vi "main.vi"() -> ()   [LabVIEW 2020]
uses:
  measure/Meas Session.ctl
  adc/ADC Session.ctl
  drivers/niScope/niScope Session.ctl
  drivers/niScope/niScope Virtual Channel Config.ctl
  drivers/niScope/niScope Virtual Channel Mode.ctl
  drivers/niScope/niScope Virtual Channel Input Z.ctl
  drivers/niScope/niScope Virtual Channel Coupling.ctl
  drivers/niScope/niScope Type.ctl
  drivers/niScope/niScope Digitizing Process Options.ctl
  drivers/niScope/niScope Data Packet.ctl
  drivers/niScope/niScope Trigger Setup.ctl
  <instrlib>/niScope/Controls/niScope trigger coupling.ctl
  <instrlib>/niScope/Controls/niScope trigger slope.ctl
  drivers/niScope/niScope Reference Clock.ctl
  drivers/DMM/3458A Digitizer Session.ctl
  drivers/DMM/3458A Virtual Channel Config.ctl
  drivers/Counter/Counter Session.ctl
  drivers/Counter/Counter Type.ctl
  drivers/AWG/AWG Session.ctl
  drivers/AWG/AWG Type.ctl
  drivers/AWG/CMI Clock Divider v2/CMI ckd2 Session.ctl
  drivers/AWG/CMI Clock Divider v2/CMI ckd2 Source Mode.ctl
  drivers/AWG/CMI Clock Divider v2/CMI ckd2 Divisor Mode.ctl
  drivers/AWG/CMI Sync V3/CMI Sync V3 session.ctl
  drivers/AWG/CMI Sync V3/Configure/CMI Sync V3 Reference Clock Source.ctl
  drivers/AWG/CMI Sync V3/Configure/CMI Sync V3 HV input Range.ctl
  drivers/AWG/CMI Sync V3/Configure/CMI Sync V3 Trigger Input Level.ctl
  drivers/AWG/CMI Sync V3/Configure/CMI Sync V3 Channel 1 Mode.ctl
  drivers/AWG/CMI Sync V3/Configure/CMI Sync V3 Channel Output Levels.ctl
  drivers/AWG/CMI Sync V3/Configure/CMI Sync V3 Channel 2 Mode.ctl
  drivers/AWG/CMI Sync V3/Configure/CMI Sync V3 Channel 3 Mode.ctl
  drivers/AWG/CMI Sync V3/Configure/CMI Sync V3 Channel 1 Divisor Entry Mode.ctl
  adc/ADC Trig Config.ctl
  adc/ADC Trig Mode Source.ctl
  adc/ADC Trig Slope.ctl
  adc/ADC Trig Coupling.ctl
  drivers/AWG/RaS HMF2500/HMF2500 Config.ctl
  drivers/DMM/3458A Sync Mode.ctl
  drivers/DMM/3458A Idn Mode.ctl
  drivers/DMM/3458A Digitizing Low Levels/Configure/Sampling Mode.ctl
  drivers/DMM/3458A Digitizing Process Options.ctl
  drivers/DMM/3458A Data Packet.ctl
  drivers/DMM/3458A Aux Record Data.ctl
  drivers/DMM/3458A Digitizing Low Levels/Configure/Level Setup.ctl
  drivers/DMM/3458A Digitizing Low Levels/Configure/First Sample Trigger.ctl
  drivers/DMM/3458A Aperture Selection Mode.ctl
  drivers/DMM/3458A Multiplexing Config.ctl
  drivers/Fluke 8588A/F8588A Low Pass Filter.ctl
  drivers/Fluke 8588A/F8588A Phase Lock.ctl
  drivers/Fluke 8588A/F8588A Coupling.ctl
  drivers/DMM/3458A Sampling Rate.ctl
  drivers/AWG/AWG Clock Setup Mode.ctl
  drivers/DMM/3458A Sample Rate Mode.ctl
  drivers/dsdll/DSDLL Session.ctl
  drivers/dsdll/dsdll/dsdll_instance.ctl
  drivers/dsdll/dsdll/dsdll_device_record.ctl
  drivers/dsdll/DSDLL Process Config.ctl
  drivers/dsdll/DSDLL Data Packet.ctl
  adc/ADC Type.ctl
  drivers/simulated_adc/SimAdc Config.ctl
  drivers/simulated_adc/SimAdc Channel Cfg.ctl
  adc/ADC On Close Action.ctl
  adc/Multiplexer/MPX Session.ctl
  adc/Multiplexer/MPX Type.ctl
  drivers/Multiplexers/Generic COM/GCOMM Session.ctl
  drivers/Multiplexers/Generic COM/GCOMM Signal.ctl
  drivers/Multiplexers/Generic COM/GCOMM Virtual Channel.ctl
  drivers/Multiplexers/Generic COM/GCOMM Logic State.ctl
  drivers/Multiplexers/Generic COM/QPMX Session.ctl
  drivers/Multiplexers/QPMX/QPMX switch mode.ctl
  drivers/Multiplexers/QPMX/QPMX polarity.ctl
  drivers/Multiplexers/Generic VISA commands/GVISA Mux Session.ctl
  drivers/Multiplexers/Generic VISA commands/GVISA Mux Path Entry.ctl
  drivers/Multiplexers/Generic VISA commands/met_serial_setup.ctl
  drivers/Agilent DSO 90000/Virtual Digitizer/KeDSO session.ctl
  drivers/Agilent DSO 90000/Virtual Digitizer/KeDSO Virtual Channel.ctl
  drivers/Agilent DSO 90000/Virtual Digitizer/KeDSO High Resolution Mode.ctl
  drivers/Agilent DSO 90000/Virtual Digitizer/KeDSO Trigger Setup.ctl
  drivers/Agilent DSO 90000/Virtual Digitizer/KeDSO Trigger Source.ctl
  drivers/Agilent DSO 90000/Public/Utility/DSO type.ctl
  drivers/cdaq/cDAQ Session.ctl
  drivers/cdaq/low_level_old/cdaq_anal_adc_command.ctl
  drivers/cdaq/low_level_old/cdaq_anal_adc_data.ctl
  drivers/cdaq/cDAQ Virtual Channel.ctl
  drivers/cdaq/cDAQ Master Clock Mode.ctl
  measure/Meas Sequence Item.ctl
  measure/Meas Sampling Configuration.ctl
  measure/processing/QWTB/Meas Proc QWTB Algorithm Parameter Data.ctl
  measure/Meas Sequence Configuration.ctl
  measure/Meas Range Mode.ctl
  measure/Meas Sampling Rate Mode.ctl
  octave/golpi/mpc/golpi_session_ref.ctl
  octave/golpi/mpc/golpi_session.ctl
  octave/golpi/GOLPI reference Type Def.ctl
  octave/golpi/Pipe Handle.ctl
  measure/processing/Meas Process Config.ctl
  measure/processing/Meas Process Mode.ctl
  measure/processing/Meas Process Raw Config.ctl
  measure/processing/Meas Process Raw Result Mode.ctl
  measure/processing/QWTB/Meas Proc QWTB Setup.ctl
  measure/processing/QWTB/Meas Proc QWTB Uncertainty Mode.ctl
  measure/processing/QWTB/Meas Proc QWTB Multicore Setup.ctl
  measure/processing/QWTB/Meas Proc QWTB Multicore Type.ctl
  measure/processing/Meas Process Time Stamp Mode.ctl
  measure/processing/QWTB/Meas Proc QWTB Exec Mode.ctl
  measure/Corrections/Corr Setup.ctl
  measure/Corrections/Corr Tranducer Item.ctl
  measure/Corrections/Corr Digitizers.ctl
  measure/Assist/Assist Panel Setup.ctl
  measure/processing/QWTB/Meas Proc QWTB View Max Dim.ctl
  measure/processing/QWTB/Meas Proc QWTB View Uncertainty Mode.ctl
  measure/processing/QWTB/Meas Proc QWTB View Group Mode.ctl
  measure/processing/QWTB/Meas Proc QWTB Viewer References.ctl
  measure/processing/QWTB/Meas Proc QWTB View Phase Mode.ctl
  measure/processing/QWTB/Meas Proc QWTB View Amplitude Mode.ctl
  server/Server Event GUI command.ctl
  server/Server Session.ctl
  varilib/SGUI Assign References Mode.ctl
  server/Server Event.ctl
  server/Server Client Request.ctl
  server/Server Event Command.ctl
  <vilib>/Utility/miscctls.llb/LVRowAndColumnTypeDef.ctl
  varilib/SGUI Assign Multiple Strings With Tags By Label.vi
  varilib/varilib.lvlib
  drivers/niScope/niScope Virtual Digitizer.lvlib
  drivers/DMM/3458A Virtual Digitizer.lvlib
  drivers/Counter/Counter.lvlib
  drivers/AWG/AWG.lvlib
  drivers/DMM/3458A Digitizing Low Levels/3458A Digitizing Low Levels.lvlib
  drivers/dsdll/DSDLL Virtual Digitizer.lvlib
  octave/golpi/mpc/GOLPI Multi Process.lvlib
  drivers/dsdll/dsdll/dsdll.lvlib
  drivers/AWG/CMI Sync V3/CMI Sync Unit V3.lvlib
  drivers/Agilent DSO 90000/Agilent 90000 Series.lvlib
  octave/golpi/GOLPI library.lvlib
  octave/golpi/LV Process library.lvlib
panel:
  out "stat4":string
  in  "btn view fft":bool
  in  "server":T1
  out "start btns":T2
  in  "server vi ref":refnum<vi>
  in  "btn srv":bool
  in  "btn qwtb calc":bool
  in  "qwtb view VI ref":refnum<vi>
  in  "exp tab":string[][](table)
  in  "btn about":bool
  out "qwtb view":T3
  in  "tc result":enum32{"RAW", "QWTB"}(tab)=enum."QWTB"
  out "str res":string caption="Result"
  in  "qwtb comment":string caption="Note:"
  in  "qwtb amp":T4 caption="Convert amplitude"
  out "qwtb meas pth":string caption="Selected measurement:"
  in  "qwtb alg sel":u16(ring) caption="Algorithm selection" items=["Current: TWM-PWRTDI", "TWM-PWRTDI"]
  in  "qwtb meas sel":u16(ring) caption="Measurement selection" items=["None", "Current", "Load from file"]
  in  "qwtb ref chn":u16(ring) caption="Ref. channel" items=["None", "L1"]
  in  "qwtb ph unit":T5 caption="Phase mode"
  out "qwtb res info":string caption="Info:"
  in  "qwtb res sel":u16(ring) caption="Result selection" items=["Current result", "Average", "RESULTS\\TWM-PWRTDI-G0001-A0001"]
  in  "qwtb maxarr":i32=10 caption="Max shown array size" min=1 max=1000 step=1
  in  "qwtb order":T6 caption="Res. order mode"
  in  "qwtb unc":T7 caption="Uncertainty display"
  in  "qwtb maxdim":T8 caption="Max. shown dimension"
  out "qwtb results table":string[][](table) caption="Results (right click to table to show actions)"
  in  "qwtb qu list":i32[](listbox) caption="Select quantities"
  in  "qwtb save comment":bool
  in  "btn set&start":bool
  in  "btn setup":bool
  in  "btn corr":bool
  in  "btn view rec":bool
  in  "golpi":T9={"GOLPI ref"={"pipe handle"={"lv_proc.dll file path"=path "", "process instance handle"=[], "debug mode"=FALSE, "debug data"=[]}, "fast read timeout [ms]"=500, "fast read settle time [ms]"=10, "fast read to multiple [ms]"=1, "max elements per input line"=100, "slow read timeout [ms]"=5000, "stdin double format specifier"="%_16e", "max elements per stdout output column"=100, "console mode bitstream"=FALSE, "bitstream first read timeout [ms]"=1000, "bitstream read timeout [ms]"=50, "struct transfer possible"=FALSE, "matlab mode"=FALSE}, "idn str"="", "octave path"=path "C:/Octave364/Octave3.6.4_gcc4.6.2/bin", "work path"=path "C:/Octave364/Octave3.6.4_gcc4.6.2/bin", "start timeout [ms]"=15000, "clr cache"=FALSE, "console"=FALSE, "binary"=FALSE, "semaphore"=refnum, "initial command"="", "exit command"="", "matlab"=FALSE, "pkg list"=[]}
  out "stat3":string
  out "stat2":string
  in  "session VI ref":refnum<vi>
  out "stat1":string
  in  "session":T13={"adc"={"niScope"={"channel cfg"=[], "sessions"=[], "multi cards"=FALSE, "channels"=0, "type"=enum."n/a", "memory [B/chn]"=0, "ext. clock [Hz]"=0.0, "samples count"=0, "use streaming"=FALSE, "proc setup"={"packet size [smpl]"=0, "current timeout [s]"=0.0, "blk2blk timeout [s]"=0.0, "event time"=timestamp(0 s since 1904-01-01), "temp sampl T [s]"=0.0, "data queue"=refnum, "stop notifier"=refnum, "proc ref"=refnum}, "sample width [B]"=0, "ranges [V]"=[], "trigger setup"={"coupling"=1, "level [V]"=0.0, "slope"=0, "mode"=enum."Immediate", "pre-trigger [%]"=0.0}, "fs [Hz]"=0.0, "bitres [bit]"=0, "clock source"=enum."VAL_NO_SOURCE"}, "3458A"={"channels"=[], "sync unit"={"VISA"="", "type"=enum."Picotest U6200A"}, "awg unit"={"type"=enum."Agilent 331xxA to 332xxA", "VISA"="", "enable 10MHz ref"=FALSE, "cmi ckd2"={"VISA"="", "clock source"=enum."Auto", "manual ref clk"=FALSE, "ref clock [Hz]"=0.0, "div mode"=enum."Set divisor directly"}, "cmi sync v3"={"VISA"="", "baud rate [bd/s]"=115200, "source"=enum."Auto", "hv range"=enum."1kV", "fsrc is fixed"=FALSE, "fsrc [Hz]"=10000000.0, "freq integ [s]"=1.0, "freq filter"=5, "trig level"=enum."TTL 5V", "chn1 mode"=enum."Source divider", "chn1 level"=enum."Positive 5V", "chn2 mode"=enum."Source divider", "chn2 level"=enum."Positive 5V", "chn2 div"=1, "chn3 mode"=enum."Chn 1 Active", "chn3 level"=enum."Positive 5V", "chn1 div entry"=enum."Calculate nearest divisor from measured fx", "chn1 dev limit [%]"=1.0, "chn1 check dev"=FALSE}, "trigger"={"source"=enum."Immediate", "slope"=enum."POS", "coupling"=enum."DC", "level [V]"=0.0, "hysteresis [V]"=0.0, "pre-trigger [%]"=0.0}, "HMF2500 cfg"={"Baud Rate"=9600, "Parity"=0, "Data Bits"=8, "Flow Control"=4}}, "sync mode"=enum."MASTER-SLAVE, MASTER clocked by TIMER", "streaming mode"=FALSE, "idn mode"=enum."Auto", "sampling mode"=enum."DCV", "sample memory [B]"=0, "proc setup"={"channel id"=0, "packet size [smpl]"=0, "current timeout [s]"=0.0, "blk2blk timeout [s]"=0.0, "event time"=timestamp(0 s since 1904-01-01), "stop notifier"=refnum, "data queues"=[], "proc refs"=[], "bus semaphore"=refnum}, "sample size [B]"=0, "sample count"=0, "aux data"={"channel id"=0, "valid?"=[], "gain [V]"=[], "timestamp [s]"=[], "Ts [s]"=0.0, "abs timestamp"=timestamp(0 s since 1904-01-01), "t [deg C]"=[], "multiplex timestamp [s]"=-1.0, "only multiplex?"=FALSE, "multiplex smpl offset"=0, "overflow?"=FALSE}, "ranges [V]"=[], "aperture [s]"=0.0, "LEVEL trigger"={"edge"=enum."POS", "level [V]"=0.0, "coupling"=enum."DC"}, "trigger mode"=enum."AUTO", "measure temp.?"=FALSE, "disp mesages"=[], "shared bus?"=FALSE, "disable display?"=FALSE, "aper mode"=enum."Manual", "aper rules"=[], "multiplex"={"cycles"=0, "delay [s]"=0.0, "enabled"=FALSE, "overhead [s]"=1.0, "tot smpls"=0, "sub-rec"=0, "overhead [%]"=0.0, "emulated"=FALSE}, "F8588 lpf"=enum."Off", "F8588 pll"=enum."Off", "F8588 couple"=enum."DC, auto", "fs"={"freq mode"=enum."fs or Ts", "fs [Hz]"=0.0, "fref [Hz]"=0.0, "mul"=0.0, "div"=0.0}, "fs mode"=enum."fs or Ts"}, "dsdll"={"dsdll"={"dsdll path"=path "", "dsdll handle"=[], "output devices"=[], "capture devices"=[]}, "channels"=0, "device id"=0, "channel idns"=[], "proc setup"={"packet size [smpl]"=0, "current timeout [s]"=0.0, "blk2blk timeout [s]"=0.0, "event time"=timestamp(0 s since 1904-01-01), "data queue"=refnum, "stop notifier"=refnum, "proc ref"=refnum}, "samples count"=0, "fs [Hz]"=0.0}, "type"=enum."niScope", "channel idn str"=[], "aux instr idn str"=[], "modified?"=FALSE, "simadc"={"channels"=[], "range [V]"=0.0, "Ts step [s]"=0.0, "time [s]"=0.0, "fs [Hz]"=0.0, "count"=0, "smpl offset"=0, "set count"=0, "bit res"=0}, "force rst?"=FALSE, "exit mode"=enum."Immediate reset", "exit dly"=0.0, "exit tmr"=timestamp(0 s since 1904-01-01), "busy?"=FALSE, "accessed?"=FALSE, "multiplex"={"Type"=enum."Dummy", "gen com ssn"={"visa"="", "primary"=enum."None", "secondary"=enum."None", "channels"=[]}, "delay before [s]"=0.0, "delay post [s]"=0.0, "sequence"=[], "enabled"=FALSE, "ref timestamp [s]"=0.0, "idn string"="", "dev niScope"="", "niScope idx"=0, "QPMX ssn"={"visa"="", "switch mode"=enum."Switched by TWM", "sequence"=[], "timing delays"=[], "polarity"=enum."Positive", "ss delay (s)"=2.0, "internal timer (s)"=1.0, "Last loaded sequence file"=path "", "startup delay (s)"=2.0}, "VISA mux ssn"={"VISA"="", "paths"=[], "idn command"="", "serial cfg"={"Baud rate"=9600, "Data bits"=8, "Parity"=0, "Stop bits"=10, "Flow control"=0, "End Mode Read"=enum."None", "End Mode Write"=enum."None", "Term character"=0, "Term enable"=FALSE}}}, "keysight dso"={"VISA"="", "channels"=[], "bw limit [Hz]"=0.0, "resolution"=enum."Basic", "trig noise reject"=enum."Normal", "N"=0, "trigger config"={"trigger source"=enum."Immediate", "trigger slope"=enum."Negative", "level [V]"=0.0, "hysteresis [V]"=0.001, "pre-trig [%]"=50}, "fs [Hz]"=0.0, "timeout stop"=timestamp(0 s since 1904-01-01), "waiting for opc"=FALSE, "fetch offset [smpl]"=0, "abs timestamp"=timestamp(0 s since 1904-01-01), "ranges [V]"=[], "decimation"=1.0, "ext ref"=FALSE, "emulate aperture"=FALSE, "model"=enum."DSO91304"}, "cdaq"={"mclk [Hz]"=12800000.0, "ADC task"="", "mclk reference"="", "fs [Hz]"=50000.0, "queue adc cmd"=refnum, "queue adc data"=refnum, "adc proc ref"=refnum, "channels"=[], "last channels"=[], "timeout"=timestamp(0 s since 1904-01-01), "N"=1000, "mclk mode"=enum."Free running", "ext mclk source"=""}, "ignore overload"=FALSE}, "sequence"=[], "sequence setup"={"group setups"=[], "rec count"=0, "range mode"=enum."Keep defaults", "fs mode"=enum."Frequency", "rng even"=0.0, "rng odd"=0.0, "folder"=path "", "name base"="", "meas id"=0, "settle [s]"=0.0, "comment"="", "avg count"=0, "fs-abs-fr fr"=0.0, "fs-abs-fr fs"=0.0, "fs-div fr"=0.0, "fs-div div"=0.0, "fs-mn fr"=0.0, "fs-mn mul"=0.0, "fs-mn div"=0.0, "fs-rat fr"=0.0, "fs-rat rat"=0.0}, "golpi"=refnum, "processing setup"={"mode"=enum."Raw", "call after avgs?"=FALSE, "calculate?"=FALSE, "raw mode"={"command"="", "result mode"=enum."Display console output (only Octave)", "res variable"=""}, "QWTB"={"QWTB path"=path "", "alg filter path"="", "alg ids"=[], "alg parameters"=[], "parsed parameters"=[], "selected alg id"="", "selected unc mode"=enum."None", "qwtb mcc"=100, "qwtb timeout"=90, "qwtb covg"=95.0, "qwtb ofs"=0, "qwtb lim data"=0, "multicore"={"jobs folder"=path "", "cores"=0, "max jobs"=0, "mode"=enum."Singlecore"}, "unc once?"=FALSE, "qwtb tstemp"=enum."Enabled (default)", "octave reset"=FALSE, "exec mode"=enum."Single-core"}}, "corrections"={"transducers"={"channels"=[], "last path"=path "", "root path"=path ""}, "digitizer"={"last path"=path "", "channel paths"=[], "channel idns"=[], "correction name"="", "channel names"=[], "folders to copy"=[], "channel valid"=[], "correction path"=path "", "correction rel path"="", "rel folders to copy"=[], "root path"=path ""}}, "assist cfg"={"P"=0, "Q"=0, "rel shift"=0.0, "ref freq"=0.0, "min fs"=0.0, "max fs tol"=0.0, "min int"=0.0, "max int"=0.0, "max err"=0.0, "max timeout"=0.0}} {"corrections"."transducers"."channels"."Phase index" min=1 step=1; "adc"."cdaq"."last channels"."Channel id" min=0 step=1; "adc"."cdaq"."channels"."Channel id" min=0 step=1; "adc"."keysight dso"."decimation" min=1.0; "adc"."keysight dso"."bw limit [Hz]" format="%#_6p"; "adc"."keysight dso"."channels"."Offset [V]" format="%#_6p"; "adc"."keysight dso"."channels"."Range [Vpk]" min=0.0 format="%#_6p"; "adc"."keysight dso"."channels"."Channel" min=1; "adc"."multiplex"."VISA mux ssn"."serial cfg"."Flow control" items=["None", "XON/XOFF", "CTS/RTS", "XON/XOFF + CTS/RTS", "DTR/DSR", "XON/XOFF + DTR/DSR"]; "adc"."multiplex"."VISA mux ssn"."serial cfg"."Stop bits" items=["1 bit"=10, "1.5 bits"=15, "2 bits"=20]; "adc"."multiplex"."VISA mux ssn"."serial cfg"."Parity" items=["None", "Odd", "Even", "Mark", "Space"]; "adc"."multiplex"."VISA mux ssn"."serial cfg"."Data bits" items=["5 bits"=5, "6 bits"=6, "7 bits"=7, "8 bits"=8]; "adc"."multiplex"."VISA mux ssn"."serial cfg"."Baud rate" items=["150 Bd"=150, "300 Bd"=300, "600 Bd"=600, "1200 Bd"=1200, "2400 Bd"=2400, "4800 Bd"=4800, "9600 Bd"=9600, "19.2 kBd"=19200, "38.4 kBd"=38400, "57.6 kBd"=57600, "115.2 kBd"=115200]; "adc"."multiplex"."QPMX ssn"."startup delay (s)" min=0.0 step=1.0; "adc"."multiplex"."QPMX ssn"."internal timer (s)" min=0.0 step=1.0; "adc"."multiplex"."QPMX ssn"."ss delay (s)" min=0.0 step=1.0; "adc"."multiplex"."QPMX ssn"."timing delays" min=1 max=255 step=1; "adc"."3458A"."awg unit"."HMF2500 cfg"."Flow Control" items=["None", "XON/XOFF", "RTS/CTS", "XON/XOFF & RTS/CTS", "DTR/DSR", "XON/XOFF & DTR/DSR"]; "adc"."3458A"."awg unit"."HMF2500 cfg"."Data Bits" items=["7"=7, "8"=8]; "adc"."3458A"."awg unit"."HMF2500 cfg"."Parity" items=["None", "Odd", "Even", "Mark", "Space"]; "adc"."3458A"."awg unit"."HMF2500 cfg"."Baud Rate" items=["300"=300, "600"=600, "1200"=1200, "2400"=2400, "4800"=4800, "9600"=9600, "19200"=19200]; "adc"."3458A"."awg unit"."cmi sync v3"."chn2 div" min=1 max=100000000 step=1; "adc"."3458A"."awg unit"."cmi sync v3"."fsrc [Hz]" format="%_8p"; "adc"."3458A"."channels"."Range [Vpk]" min=0.0; "adc"."niScope"."trigger setup"."pre-trigger [%]" format="%.2f"; "adc"."niScope"."trigger setup"."level [V]" format="%.2f"; "adc"."niScope"."trigger setup"."coupling" items=["AC"=0, "DC"=1, "HF Reject"=3, "LF Reject"=4, "AC Plus HF Reject"=1001]; "adc"."niScope"."channel cfg"."Range [Vpk]" min=0.0; "adc"."niScope"."channel cfg"."Channel" min=0}
  in  "btn stop":bool
  in  "btn start":bool
  out "error":errorcluster
  in  "btn exit":bool
  in  "btn cfg adc":bool
  in  "btn cfg octave":bool
  # "ADC:"
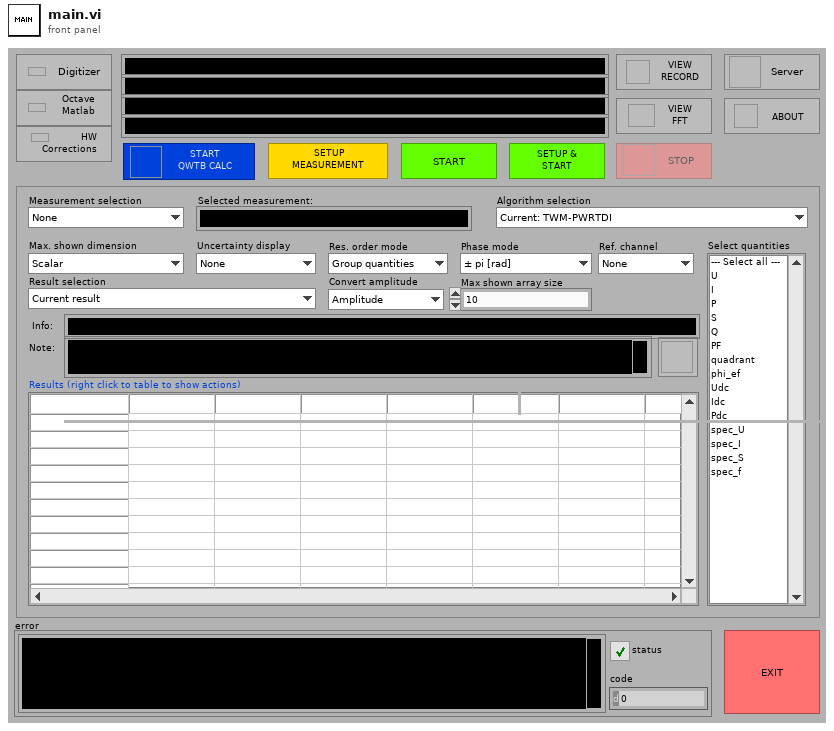
[diagram p1: front panel]
types:
  T1 = typedef "Server Session.ctl" = cluster{"cmd event":variant, "answer event":variant}
  T2 = typedef "Server Event GUI command.ctl" = cluster{"start":bool, "setup":bool, "setup&start":bool}
  T3 = typedef "Meas Proc QWTB Viewer References.ctl" = cluster{"tc result":refnum<vi>, "qwtb results tbl":refnum<vi>, "qwtb maxdim":refnum<vi>, "qwtb unc":refnum<vi>, "qwtb order":refnum<vi>, "qwtb maxarr":refnum<vi>, "qwtb res sel":refnum<vi>, "qwtb res info":refnum<vi>, "descriptions":string[], "var names":string[], "channel indexes":i32[], "qwtb ref chn":refnum<vi>, "qwtb ph unit":refnum<vi>, "qwtb alg sel":refnum<vi>, "qwtb meas sel":refnum<vi>, "qwtb ssn info":refnum<vi>, "last session (man)":path, "qwtb qu list":refnum<vi>, "matrix":dbl[][], "comment":string, "qwtb comment":refnum<vi>, "last session":path, "qwtb amp":refnum<vi>}
  T4 = typedef "Meas Proc QWTB View Amplitude Mode.ctl" = enum16{"Amplitude", "Effective", "amp. * sqrt(3)", "amp. / sqrt(3)", "eff. * sqrt(3)", "eff. / sqrt(3)", "Peak-Peak", "dB", "dBmV (dBmA)", "dBuV (dBuA)"}
  T5 = typedef "Meas Proc QWTB View Phase Mode.ctl" = enum16{"± pi [rad]", "0 - 2*pi [rad]", "±180 [deg]", "0 - 360 [deg]"}
  T6 = typedef "Meas Proc QWTB View Group Mode.ctl" = enum16{"Group quantities", "Group phases"}
  T7 = typedef "Meas Proc QWTB View Uncertainty Mode.ctl" = enum16{"None", "val ± unc", "[val; unc]"}
  T8 = typedef "Meas Proc QWTB View Max Dim.ctl" = enum16{"Scalar", "Vector", "Matrix"}
  T9 = typedef "GOLPI Multi Process.lvlib/golpi_session.ctl" = cluster{"GOLPI ref":T10, "idn str":string, "octave path":path, "work path":path, "start timeout [ms]":u32, "clr cache":bool, "console":bool, "binary":bool, "semaphore":T12, "initial command":string, "exit command":string, "matlab":bool, "pkg list":string[]}
  T10 = typedef "GOLPI library.lvlib/GOLPI reference Type Def.ctl" = cluster{"pipe handle":T11, "fast read timeout [ms]":u32, "fast read settle time [ms]":u32, "fast read to multiple [ms]":u32, "max elements per input line":u32, "slow read timeout [ms]":u32, "stdin double format specifier":string, "max elements per stdout output column":u32, "console mode bitstream":bool, "bitstream first read timeout [ms]":u32, "bitstream read timeout [ms]":u32, "struct transfer possible":bool, "matlab mode":bool}
  T11 = typedef "LV Process library.lvlib/Pipe Handle.ctl" = cluster{"lv_proc.dll file path":path, "process instance handle":u32[], "debug mode":bool, "debug data":cluster{"time":timestamp, "stdin":bool, "data":string}[]}
  T12 = typedef "Semaphore RefNum" = refnum<k1>
  T13 = typedef "Meas Session.ctl" = cluster{"adc":T14, "sequence":T93[], "sequence setup":T96, "golpi":T99, "processing setup":T100, "corrections":T110, "assist cfg":T113}
  T14 = typedef "ADC Session.ctl" = cluster{"niScope":T15, "3458A":T26, "dsdll":T64, "type":T68, "channel idn str":string[], "aux instr idn str":string[], "modified?":bool, "simadc":T69, "force rst?":bool, "exit mode":T71, "exit dly":dbl, "exit tmr":timestamp, "busy?":bool, "accessed?":bool, "multiplex":T72, "keysight dso":T84, "cdaq":T90, "ignore overload":bool}
  T15 = typedef "niScope Virtual Digitizer.lvlib/niScope Session.ctl" = cluster{"channel cfg":T16[], "sessions":refnum<k20>[], "multi cards":bool, "channels":i32, "type":T20, "memory [B/chn]":i32, "ext. clock [Hz]":dbl, "samples count":i64, "use streaming":bool, "proc setup":T21, "sample width [B]":i32, "ranges [V]":dbl[], "trigger setup":T22, "fs [Hz]":dbl, "bitres [bit]":i32, "clock source":T25}
  T16 = typedef "niScope Virtual Digitizer.lvlib/niScope Virtual Channel Config.ctl" = cluster{"Address":refnum<k15>, "Channel":i32, "Mode":T17, "Input Z":T18, "Coupling":T19, "Range [Vpk]":dbl, "btn clr":bool, "btn up":bool, "btn down":bool}
  T17 = typedef "niScope Virtual Digitizer.lvlib/niScope Virtual Channel Mode.ctl" = enum16{"Single ended", "Unbal. differential", "Differential"}
  T18 = typedef "niScope Virtual Digitizer.lvlib/niScope Virtual Channel Input Z.ctl" = enum16{"1 MOhm", "50 Ohm"}
  T19 = typedef "niScope Virtual Digitizer.lvlib/niScope Virtual Channel Coupling.ctl" = enum16{"AC", "DC", "GND"}
  T20 = typedef "niScope Virtual Digitizer.lvlib/niScope Type.ctl" = enum16{"n/a", "5922"}
  T21 = typedef "niScope Virtual Digitizer.lvlib/niScope Digitizing Process Options.ctl" = cluster{"packet size [smpl]":i64, "current timeout [s]":dbl, "blk2blk timeout [s]":dbl, "event time":timestamp, "temp sampl T [s]":dbl, "data queue":refnum<queue>, "stop notifier":refnum<notifier>, "proc ref":refnum<vi>}
  T22 = typedef "niScope Virtual Digitizer.lvlib/niScope Trigger Setup.ctl" = cluster{"coupling":T23, "level [V]":dbl, "slope":T24, "mode":enum16{"Immediate", "External", "Level"}, "pre-trigger [%]":dbl}
  T23 = typedef "niScope trigger coupling.ctl" = u16
  T24 = typedef "niScope trigger slope.ctl" = i32
  T25 = typedef "niScope Virtual Digitizer.lvlib/niScope Reference Clock.ctl" = enum16{"VAL_NO_SOURCE", "VAL_CLK_IN", "VAL_PXI_CLOCK", "VAL_EXTERNAL"}
  T26 = typedef "3458A Virtual Digitizer.lvlib/3458A Digitizer Session.ctl" = cluster{"channels":T27[], "sync unit":T28, "awg unit":T30, "sync mode":T49, "streaming mode":bool, "idn mode":T50, "sampling mode":T51, "sample memory [B]":i32, "proc setup":T52, "sample size [B]":i32, "sample count":i32, "aux data":T53, "ranges [V]":dbl[], "aperture [s]":dbl, "LEVEL trigger":T54, "trigger mode":T55, "measure temp.?":bool, "disp mesages":string[], "shared bus?":bool, "disable display?":bool, "aper mode":T56, "aper rules":dbl[][], "multiplex":T57, "F8588 lpf":T58, "F8588 pll":T59, "F8588 couple":T60, "fs":T61, "fs mode":T63}
  T27 = typedef "3458A Virtual Digitizer.lvlib/3458A Virtual Channel Config.ctl" = cluster{"VISA":refnum<visa-resource-name>, "Range [Vpk]":dbl, "btn clr":bool, "btn up":bool, "btn down":bool, "F8588":bool, "F8588 guard":bool}
  T28 = typedef "Counter.lvlib/Counter Session.ctl" = cluster{"VISA":refnum<visa-resource-name>, "type":T29}
  T29 = typedef "Counter.lvlib/Counter Type.ctl" = enum16{"Picotest U6200A", "dummy"}
  T30 = typedef "AWG.lvlib/AWG Session.ctl" = cluster{"type":T31, "VISA":refnum<visa-resource-name>, "enable 10MHz ref":bool, "cmi ckd2":T32, "cmi sync v3":T35, "trigger":T44, "HMF2500 cfg":T48}
  T31 = typedef "AWG.lvlib/AWG Type.ctl" = enum16{"Agilent 331xxA to 332xxA", "Agilent 335xxA to 336xxA", "Tektronix AFG3101C", "R&S HMF25xx", "CMI Clock Divider v2", "CMI Sync Unit V3", "dummy"}
  T32 = typedef "AWG.lvlib/CMI ckd2 Session.ctl" = cluster{"VISA":refnum<visa-resource-name>, "clock source":T33, "manual ref clk":bool, "ref clock [Hz]":dbl, "div mode":T34}
  T33 = typedef "AWG.lvlib/CMI ckd2 Source Mode.ctl" = enum16{"Auto", "LF clock", "HF clock", "Internal"}
  T34 = typedef "AWG.lvlib/CMI ckd2 Divisor Mode.ctl" = enum16{"Set divisor directly", "Set divisor by frequency"}
  T35 = typedef "AWG.lvlib/CMI Sync Unit V3.lvlib/CMI Sync V3 session.ctl" = cluster{"VISA":refnum<visa-resource-name>, "baud rate [bd/s]":i32, "source":T36, "hv range":T37, "fsrc is fixed":bool, "fsrc [Hz]":dbl, "freq integ [s]":dbl, "freq filter":i32, "trig level":T38, "chn1 mode":T39, "chn1 level":T40, "chn2 mode":T41, "chn2 level":T40, "chn2 div":i32, "chn3 mode":T42, "chn3 level":T40, "chn1 div entry":T43, "chn1 dev limit [%]":dbl, "chn1 check dev":bool}
  T36 = typedef "AWG.lvlib/CMI Sync Unit V3.lvlib/CMI Sync V3 Reference Clock Source.ctl" = enum16{"Auto", "Internal", "Logic", "Sine", "HV"}
  T37 = typedef "AWG.lvlib/CMI Sync Unit V3.lvlib/CMI Sync V3 HV input Range.ctl" = enum16{"10V", "60V", "250V", "1kV"}
  T38 = typedef "AWG.lvlib/CMI Sync Unit V3.lvlib/CMI Sync V3 Trigger Input Level.ctl" = enum16{"LVCMOS 3V3", "TTL 5V"}
  T39 = typedef "AWG.lvlib/CMI Sync Unit V3.lvlib/CMI Sync V3 Channel 1 Mode.ctl" = enum16{"Source divider", "DDS absolute", "DDS ratio", "DDS ratio M/N"}
  T40 = typedef "AWG.lvlib/CMI Sync Unit V3.lvlib/CMI Sync V3 Channel Output Levels.ctl" = enum16{"Positive 3V3", "Negative 3V3", "Positive 5V", "Negative 5V"}
  T41 = typedef "AWG.lvlib/CMI Sync Unit V3.lvlib/CMI Sync V3 Channel 2 Mode.ctl" = enum16{"Source divider", "Chn 1 divide"}
  T42 = typedef "AWG.lvlib/CMI Sync Unit V3.lvlib/CMI Sync V3 Channel 3 Mode.ctl" = enum16{"Chn 1 Active", "Chn 2 Active", "Chn 1 Trigger", "Chn 2 Trigger", "Gate", "PPS", "10MHz"}
  T43 = typedef "AWG.lvlib/CMI Sync Unit V3.lvlib/CMI Sync V3 Channel 1 Divisor Entry Mode.ctl" = enum16{"Set divisor directly", "Calculate nearest divisor from measured fx"}
  T44 = typedef "ADC Trig Config.ctl" = cluster{"source":T45, "slope":T46, "coupling":T47, "level [V]":dbl, "hysteresis [V]":dbl, "pre-trigger [%]":dbl}
  T45 = typedef "ADC Trig Mode Source.ctl" = enum16{"Immediate", "External", "Level"}
  T46 = typedef "ADC Trig Slope.ctl" = enum16{"POS", "NEG"}
  T47 = typedef "ADC Trig Coupling.ctl" = enum16{"DC", "AC"}
  T48 = typedef "AWG.lvlib/HMF2500 Config.ctl" = cluster{"Baud Rate":u32, "Parity":u16, "Data Bits":u16, "Flow Control":u16}
  T49 = typedef "3458A Virtual Digitizer.lvlib/3458A Sync Mode.ctl" = enum16{"MASTER-SLAVE, MASTER clocked by TIMER", "MASTER-SLAVE, MASTER clocked by AWG", "ALL clocked by AWG", "MASTER-SLAVE, ALL clocked by TIMER", "ALL clocked by AWG with DFLL"}
  T50 = typedef "3458A Virtual Digitizer.lvlib/3458A Idn Mode.ctl" = enum16{"Auto", "Sequential (chn A, chn B, ...)", "From calibration string"}
  T51 = typedef "3458A Virtual Digitizer.lvlib/3458A Digitizing Low Levels.lvlib/Sampling Mode.ctl" = enum16{"DCV", "DSDC", "DSAC"}
  T52 = typedef "3458A Virtual Digitizer.lvlib/3458A Digitizing Process Options.ctl" = cluster{"channel id":i32, "packet size [smpl]":i32, "current timeout [s]":dbl, "blk2blk timeout [s]":dbl, "event time":timestamp, "stop notifier":refnum<notifier>, "data queues":refnum<queue>[], "proc refs":refnum<vi>[], "bus semaphore":T12}
  T53 = typedef "3458A Virtual Digitizer.lvlib/3458A Aux Record Data.ctl" = cluster{"channel id":i32, "valid?":bool[], "gain [V]":dbl[], "timestamp [s]":dbl[], "Ts [s]":dbl, "abs timestamp":timestamp, "t [deg C]":dbl[], "multiplex timestamp [s]":dbl, "only multiplex?":bool, "multiplex smpl offset":i64, "overflow?":bool}
  T54 = typedef "3458A Virtual Digitizer.lvlib/3458A Digitizing Low Levels.lvlib/Level Setup.ctl" = cluster{"edge":enum16{"POS", "NEG"}, "level [V]":dbl, "coupling":enum16{"DC", "AC"}}
  T55 = typedef "3458A Virtual Digitizer.lvlib/3458A Digitizing Low Levels.lvlib/First Sample Trigger.ctl" = enum16{"AUTO", "EXT", "SYN", "SGL", "HOLD", "LEVEL"}
  T56 = typedef "3458A Virtual Digitizer.lvlib/3458A Aperture Selection Mode.ctl" = enum16{"Manual", "Maximum", "Table"}
  T57 = typedef "3458A Virtual Digitizer.lvlib/3458A Multiplexing Config.ctl" = cluster{"cycles":i32, "delay [s]":dbl, "enabled":bool, "overhead [s]":dbl, "tot smpls":i64, "sub-rec":i32, "overhead [%]":dbl, "emulated":bool}
  T58 = typedef "F8588A Low Pass Filter.ctl" = enum16{"Off", "100 kHz", "3 MHz"}
  T59 = typedef "F8588A Phase Lock.ctl" = enum16{"Off", "1 MHz", "10 MHz"}
  T60 = typedef "F8588A Coupling.ctl" = enum16{"AC, 1 MOhm", "AC, 10 MOhm", "DC, 1 MOhm", "DC, 10 MOhm", "DC, auto"}
  T61 = typedef "3458A Virtual Digitizer.lvlib/3458A Sampling Rate.ctl" = cluster{"freq mode":T62, "fs [Hz]":dbl, "fref [Hz]":dbl, "mul":dbl, "div":dbl}
  T62 = typedef "AWG.lvlib/AWG Clock Setup Mode.ctl" = enum16{"fs or Ts", "fs or Ts with fref", "fref/N", "fref*M/N", "fref*Ratio"}
  T63 = typedef "3458A Sample Rate Mode.ctl" = enum16{"fs or Ts", "fs*M/N"}
  T64 = typedef "DSDLL Virtual Digitizer.lvlib/DSDLL Session.ctl" = cluster{"dsdll":T65, "channels":i32, "device id":i32, "channel idns":string[], "proc setup":T67, "samples count":i32, "fs [Hz]":dbl}
  T65 = typedef "dsdll.lvlib/dsdll_instance.ctl" = cluster{"dsdll path":path, "dsdll handle":u8[], "output devices":T66[], "capture devices":T66[]}
  T66 = typedef "dsdll.lvlib/dsdll_device_record.ctl" = cluster{"guid":u8[], "name":string}
  T67 = typedef "DSDLL Virtual Digitizer.lvlib/DSDLL Process Config.ctl" = cluster{"packet size [smpl]":i32, "current timeout [s]":dbl, "blk2blk timeout [s]":dbl, "event time":timestamp, "data queue":refnum<queue>, "stop notifier":refnum<notifier>, "proc ref":refnum<vi>}
  T68 = typedef "ADC Type.ctl" = enum16{"niScope", "3458A", "DirectSound DLL", "Keysight DSO", "cDAQ ADC", "dummy"}
  T69 = typedef "SimAdc Config.ctl" = cluster{"channels":T70[], "range [V]":dbl, "Ts step [s]":dbl, "time [s]":dbl, "fs [Hz]":dbl, "count":i64, "smpl offset":i64, "set count":i64, "bit res":i32}
  T70 = typedef "SimAdc Channel Cfg.ctl" = cluster{"harmonics":dbl[][], "btn clear":bool, "noise":dbl, "fundamental [Hz]":dbl}
  T71 = typedef "ADC On Close Action.ctl" = enum16{"Immediate reset", "Delayed reset"}
  T72 = typedef "MPX Session.ctl" = cluster{"Type":T73, "gen com ssn":T74, "delay before [s]":dbl, "delay post [s]":dbl, "sequence":string[], "enabled":bool, "ref timestamp [s]":dbl, "idn string":string, "dev niScope":refnum<k15>, "niScope idx":i32, "QPMX ssn":T78, "VISA mux ssn":T81}
  T73 = typedef "MPX Type.ctl" = enum16{"Dummy", "Generic - COM port", "Generic - niScope PFI", "Generic - VISA commands", "QPMX"}
  T74 = typedef "GCOMM Session.ctl" = cluster{"visa":refnum<visa-resource-name>, "primary":T75, "secondary":T75, "channels":T76[]}
  T75 = typedef "GCOMM Signal.ctl" = enum16{"None", "DTR", "RTS"}
  T76 = typedef "GCOMM Virtual Channel.ctl" = cluster{"Primary:":T77, "Secondary:":T77, "btn clr":bool, "btn up":bool, "btn down":bool, "Tag:":string}
  T77 = typedef "GCOMM Logic State.ctl" = enum16{"OFF", "ON"}
  T78 = typedef "QPMX Session.ctl" = cluster{"visa":refnum<visa-resource-name>, "switch mode":T79, "sequence":bool[][], "timing delays":u32[], "polarity":T80, "ss delay (s)":dbl, "internal timer (s)":dbl, "Last loaded sequence file":path, "startup delay (s)":dbl}
  T79 = typedef "QPMX switch mode.ctl" = enum16{"Switched by TWM", "Switched by external clock", "Switched by internal clock"}
  T80 = typedef "QPMX polarity.ctl" = enum16{"Positive", "Negative"}
  T81 = typedef "GVISA Mux Session.ctl" = cluster{"VISA":refnum<visa-resource-name>, "paths":T82[], "idn command":string, "serial cfg":T83}
  T82 = typedef "GVISA Mux Path Entry.ctl" = cluster{"Tag:":string, "Command:":string, "btn clr":bool, "btn up":bool, "btn down":bool}
  T83 = typedef "met_serial_setup.ctl" = cluster{"Baud rate":i32, "Data bits":i32, "Parity":i32, "Stop bits":i32, "Flow control":i32, "End Mode Read":enum16{"None", "Last Bit", "TermChar"}, "End Mode Write":enum16{"None", "Last Bit", "TermChar"}, "Term character":u8, "Term enable":bool}
  T84 = typedef "KeDSO session.ctl" = cluster{"VISA":refnum<visa-resource-name>, "channels":T85[], "bw limit [Hz]":dbl, "resolution":T86, "trig noise reject":enum16{"Normal", "High Sensitivity"}, "N":i64, "trigger config":T87, "fs [Hz]":dbl, "timeout stop":timestamp, "waiting for opc":bool, "fetch offset [smpl]":i64, "abs timestamp":timestamp, "ranges [V]":dbl[], "decimation":dbl, "ext ref":bool, "emulate aperture":bool, "model":T89}
  T85 = typedef "KeDSO Virtual Channel.ctl" = cluster{"Channel":i32, "Range [Vpk]":dbl, "btn clr":bool, "btn up":bool, "btn down":bool, "Offset [V]":dbl, "Coupling":enum16{"DC", "DC50", "AC", "LFR1"}, "bw limit enab":bool}
  T86 = typedef "KeDSO High Resolution Mode.ctl" = enum16{"Basic", "High-res AUTO", "Min. 9-bits", "Min. 10-bits", "Min. 11-bits", "Min. 12-bits", "Fixed 11-bits", "Fixed 12-bits", "Fixed 13-bits", "Fixed 14-bits", "Fixed 15-bits", "Fixed 16-bits"}
  T87 = typedef "KeDSO Trigger Setup.ctl" = cluster{"trigger source":T88, "trigger slope":enum16{"Negative", "Positive", "Either"}, "level [V]":dbl, "hysteresis [V]":dbl, "pre-trig [%]":i32}
  T88 = typedef "KeDSO Trigger Source.ctl" = enum16{"Immediate", "Level", "AUX"}
  T89 = typedef "Agilent 90000 Series.lvlib/DSO type.ctl" = enum16{"DSO91304", "DSO91204", "DSO90804", "DSO90604", "DSO90404", "DSO90254", "DSA91304", "DSA91204", "DSA90804", "DSA90604", "DSA90404", "DSA90254", "DSO9104", "DSO9254", "DSO9404", "MSO9104", "MSO9254", "MSO9404", "MSO9064", "DSO9064", "DSOX91604", "DSOX92004", "DSOX92504", "DSOX92804", "DSOX93204", "DSO93004", "DSO9024H", "DSO9054H", "DSO9104H", "DSO9204H", "DSOS054A", "DSOS104A", "DSOS204A", "DSOS254A", "DSOS404A", "DSOS604A", "DSOS804A", "MSOS054A", "MSOS104A", "MSOS204A", "MSOS254A", "MSOS404A", "MSOS604A", "MSOS804A", "DSAX96204Q", "DSOX96204Q", "DSAX95004Q", "DSOX95004Q", "DSAX93304Q", "DSOX93304Q", "DSAX92504Q", "DSOX92504Q", "DSAX92004Q", "DSOX92004Q"}
  T90 = typedef "cDAQ Session.ctl" = cluster{"mclk [Hz]":dbl, "ADC task":refnum<k21>, "mclk reference":string, "fs [Hz]":dbl, "queue adc cmd":refnum<queue>, "queue adc data":refnum<queue>, "adc proc ref":refnum<vi>, "channels":T91[], "last channels":T91[], "timeout":timestamp, "N":i32, "mclk mode":T92, "ext mclk source":tag}
  T91 = typedef "cDAQ Virtual Channel.ctl" = cluster{"Device":tag, "Channel id":i32, "btn clr":bool, "btn up":bool, "btn down":bool}
  T92 = typedef "cDAQ Master Clock Mode.ctl" = enum16{"Free running", "Export master clock", "Import master clock"}
  T93 = typedef "Meas Sequence Item.ctl" = cluster{"config":T94, "data file path":path, "header file path":path, "group id":i32, "rec id":i32, "group done?":bool, "adc modified?":bool, "source modified?":bool, "progress [%]":dbl, "groups cnt":i32, "rec cnt":i32, "data file relative path":string, "meas root path":path, "calculate?":bool, "comment":string, "avg cnt":i32}
  T94 = typedef "Meas Sampling Configuration.ctl" = cluster{"count [smpl]":i64, "aperture [s]":dbl, "trigger":T44, "ranges [Vpk]":dbl[], "QWTB parameters":T95[], "sampling rate":T61}
  T95 = typedef "Meas Proc QWTB Algorithm Parameter Data.ctl" = cluster{"name":string, "numerics":dbl[], "strings":string[]}
  T96 = typedef "Meas Sequence Configuration.ctl" = cluster{"group setups":T94[], "rec count":i32, "range mode":T97, "fs mode":T98, "rng even":dbl, "rng odd":dbl, "folder":path, "name base":string, "meas id":i32, "settle [s]":dbl, "comment":string, "avg count":i32, "fs-abs-fr fr":dbl, "fs-abs-fr fs":dbl, "fs-div fr":dbl, "fs-div div":dbl, "fs-mn fr":dbl, "fs-mn mul":dbl, "fs-mn div":dbl, "fs-rat fr":dbl, "fs-rat rat":dbl}
  T97 = typedef "Meas Range Mode.ctl" = enum16{"Keep defaults", "Set All channels", "Set Odd and Even channels"}
  T98 = typedef "Meas Sampling Rate Mode.ctl" = enum16{"Frequency", "Period"}
  T99 = typedef "GOLPI Multi Process.lvlib/golpi_session_ref.ctl" = refnum<vi>
  T100 = typedef "Meas Process Config.ctl" = cluster{"mode":T101, "call after avgs?":bool, "calculate?":bool, "raw mode":T102, "QWTB":T104}
  T101 = typedef "Meas Process Mode.ctl" = enum16{"Raw", "QWTB"}
  T102 = typedef "Meas Process Raw Config.ctl" = cluster{"command":string, "result mode":T103, "res variable":string}
  T103 = typedef "Meas Process Raw Result Mode.ctl" = enum16{"Display console output (only Octave)", "Display string variable", "Display result file %respath%"}
  T104 = typedef "Meas Proc QWTB Setup.ctl" = cluster{"QWTB path":path, "alg filter path":string, "alg ids":string[], "alg parameters":string[], "parsed parameters":T95[], "selected alg id":string, "selected unc mode":T105, "qwtb mcc":i32, "qwtb timeout":i32, "qwtb covg":dbl, "qwtb ofs":i64, "qwtb lim data":i64, "multicore":T106, "unc once?":bool, "qwtb tstemp":T108, "octave reset":bool, "exec mode":T109}
  T105 = typedef "Meas Proc QWTB Uncertainty Mode.ctl" = enum16{"None", "GUF", "Monte Carlo"}
  T106 = typedef "Meas Proc QWTB Multicore Setup.ctl" = cluster{"jobs folder":path, "cores":i32, "max jobs":i32, "mode":T107}
  T107 = typedef "Meas Proc QWTB Multicore Type.ctl" = enum16{"Singlecore", "Multicore", "Multistation"}
  T108 = typedef "Meas Process Time Stamp Mode.ctl" = enum16{"Enabled (default)", "Disabled", "Relative to 1. record"}
  T109 = typedef "Meas Proc QWTB Exec Mode.ctl" = enum16{"Single-core", "Parallel Record Processing"}
  T110 = typedef "Corr Setup.ctl" = cluster{"transducers":cluster{"channels":T111[], "last path":path, "root path":path}, "digitizer":T112}
  T111 = typedef "Corr Tranducer Item.ctl" = cluster{"Path":path, "Ratio:":string, "Name:":string, "btn rem":bool, "btn up":bool, "btn down":bool, "s.n.:":string, "btn open":bool, "ratio o/i":dbl, "chn hi":u16, "chn lo":u16, "Phase index":i32, "btn edit":bool, "mpx chn":u16, "btn vdx1":bool, "btn csx1":bool, "invert":bool}
  T112 = typedef "Corr Digitizers.ctl" = cluster{"last path":path, "channel paths":path[], "channel idns":string[], "correction name":string, "channel names":string[], "folders to copy":path[], "channel valid":bool[], "correction path":path, "correction rel path":string, "rel folders to copy":string[], "root path":path}
  T113 = typedef "Assist Panel Setup.ctl" = cluster{"P":i32, "Q":i32, "rel shift":dbl, "ref freq":dbl, "min fs":dbl, "max fs tol":dbl, "min int":dbl, "max int":dbl, "max err":dbl, "max timeout":dbl}
  T114 = typedef "varilib.lvlib/SGUI Assign References Mode.ctl" = enum16{"Add to stack", "Overwrite", "Release last", "Release ID"}
  T115 = typedef "Server Event Command.ctl" = enum16{"None", "Restart", "Identify", "Set measurement", "Start", "Get status", "Get result", "Stop", "Set corrections", "Get algorithm info", "ADC selfcal", "Get version", "Define Multiplexer Paths", "Define Multiplexer Sequence", "Define QPMX"}
  T116 = typedef "Server Event.ctl" = cluster{"client request":T117, "command":T115}
  T117 = typedef "Server Client Request.ctl" = cluster{"info data":string, "answer handle":i32}
  T118 = enum8{"Enabled", "Disabled", "Disabled and Grayed Out"}
  T119 = typedef "Meas Proc QWTB Plot Config.ctl" = cluster{"X-axis style":T120, "Y-axis style":T120, "Show legend":T121, "Grid on":bool, "Box on":bool, "show all chn":bool}
  T120 = typedef "Meas Proc QWTB Plot Scale Mode.ctl" = enum16{"Linear", "Log"}
  T121 = typedef "Meas Proc QWTB Plot Legend.ctl" = enum16{"None", "Best", "North", "South", "East", "West", "NorthEast", "NorthWest", "SouthEast", "SouthWest"}
  T122 = typedef "LVRowAndColumnTypeDef.ctl" = cluster{"Row":i32, "Column":i32}
  T123 = cluster{"channels":T111[], "last path":path, "root path":path}
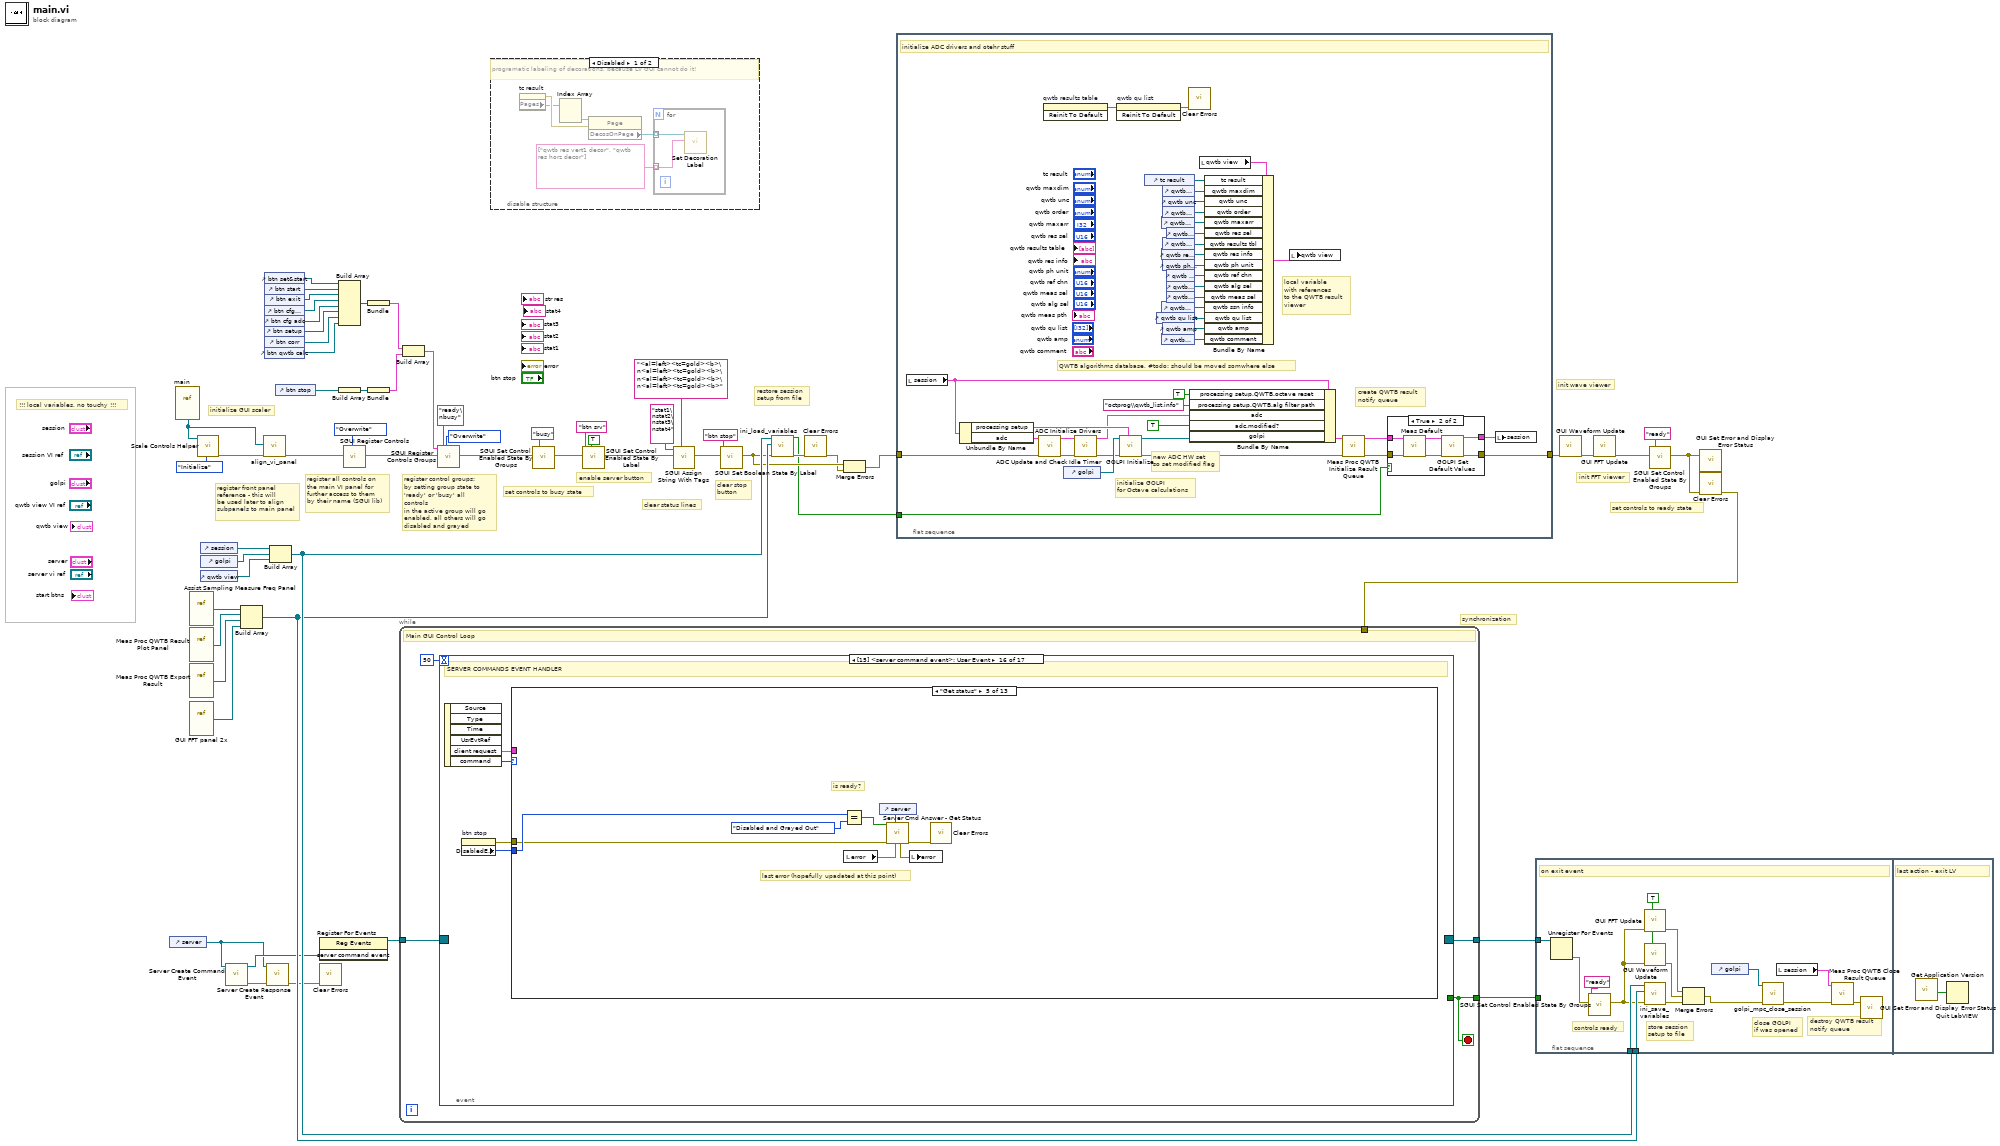
[diagram p0: block diagram]
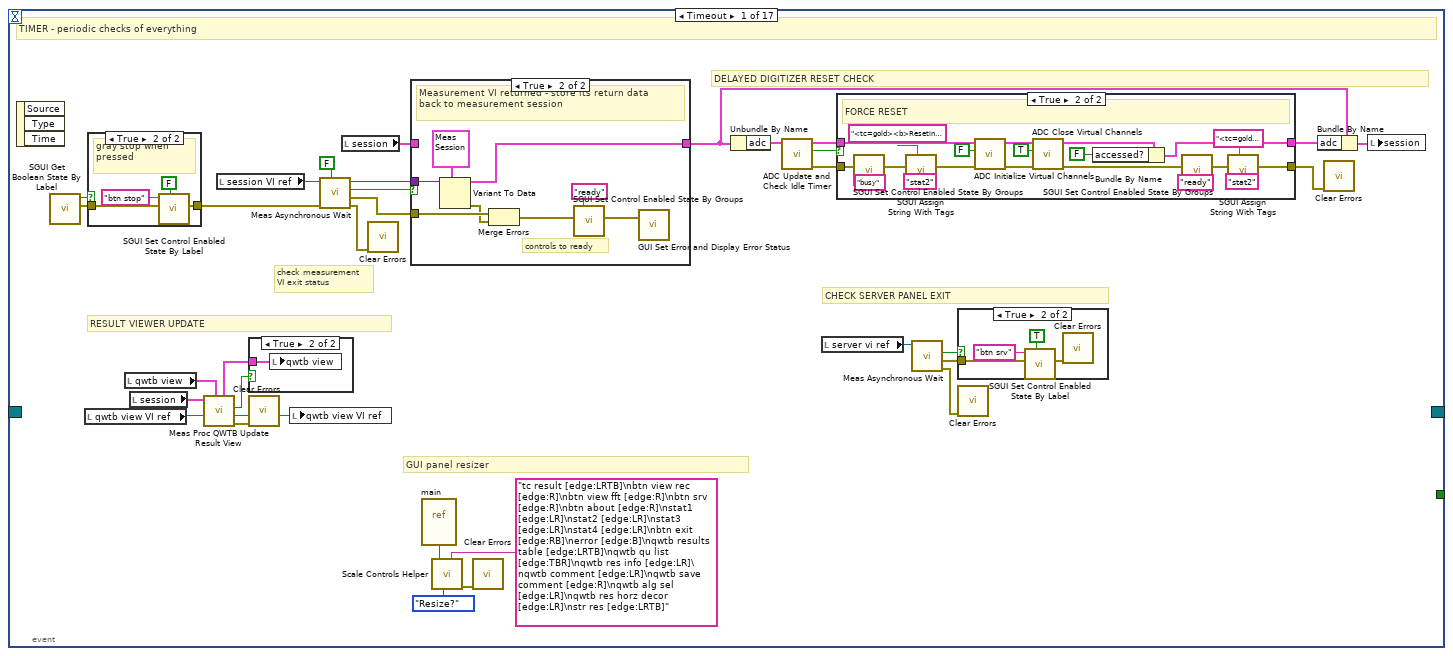
[diagram p4: hidden frame]
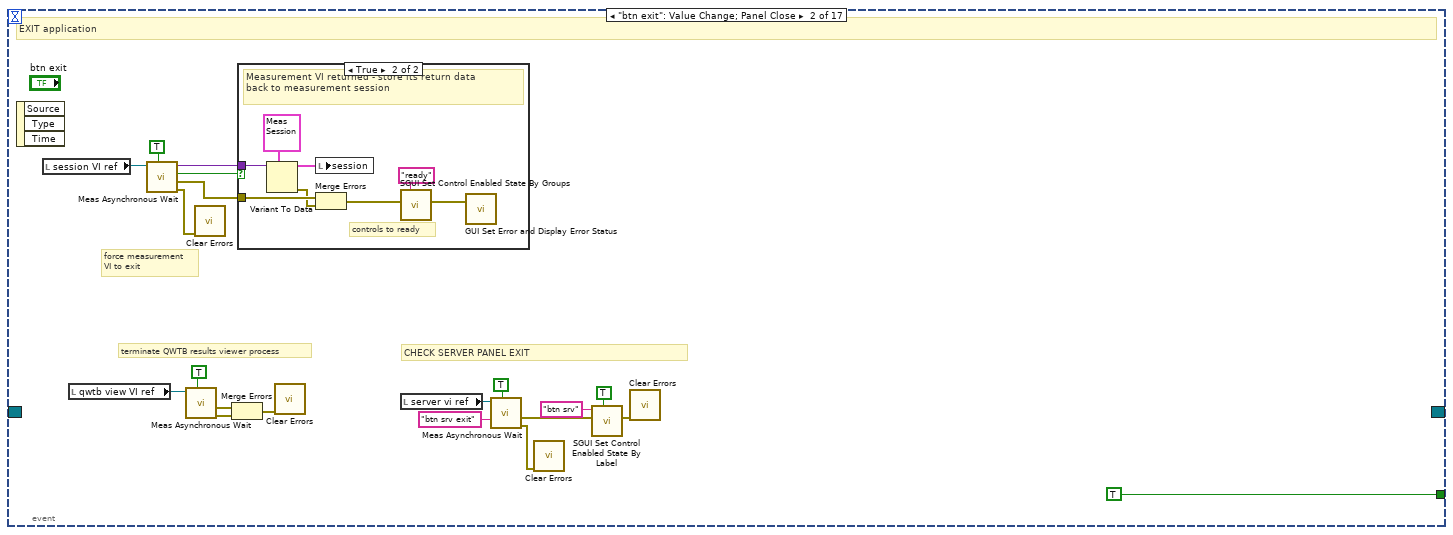
[diagram p10: hidden frame]
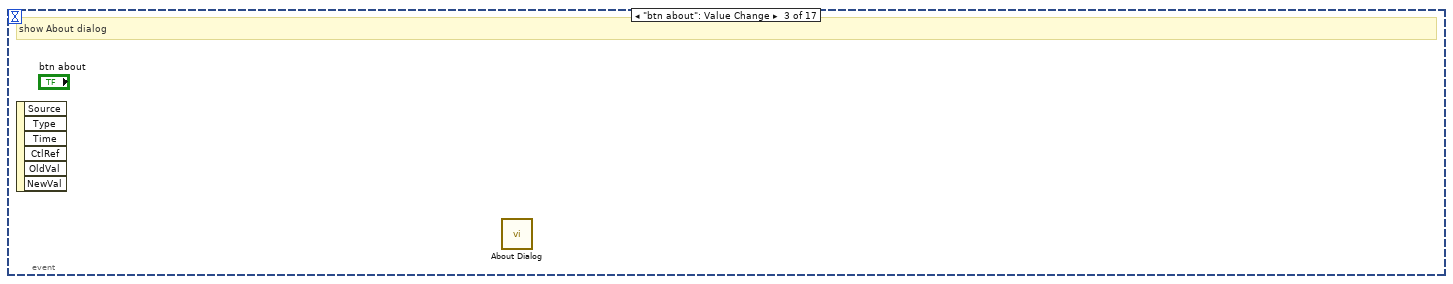
[diagram p12: hidden frame]
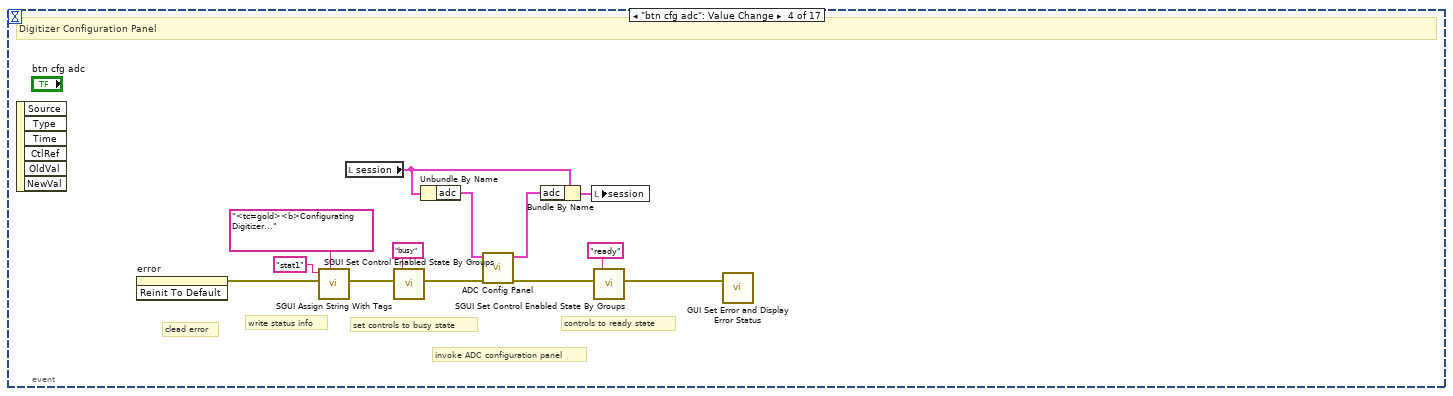
[diagram p13: hidden frame]
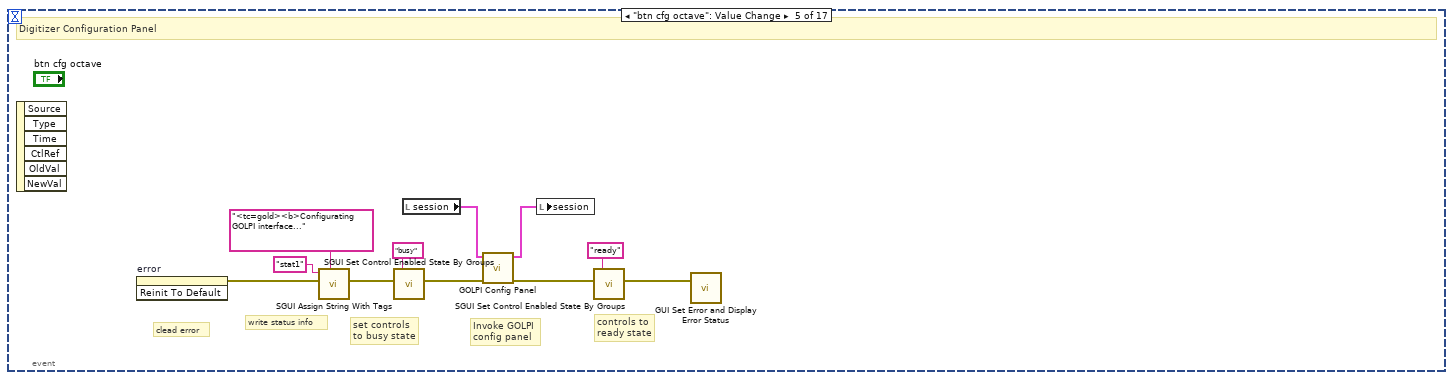
[diagram p14: hidden frame]
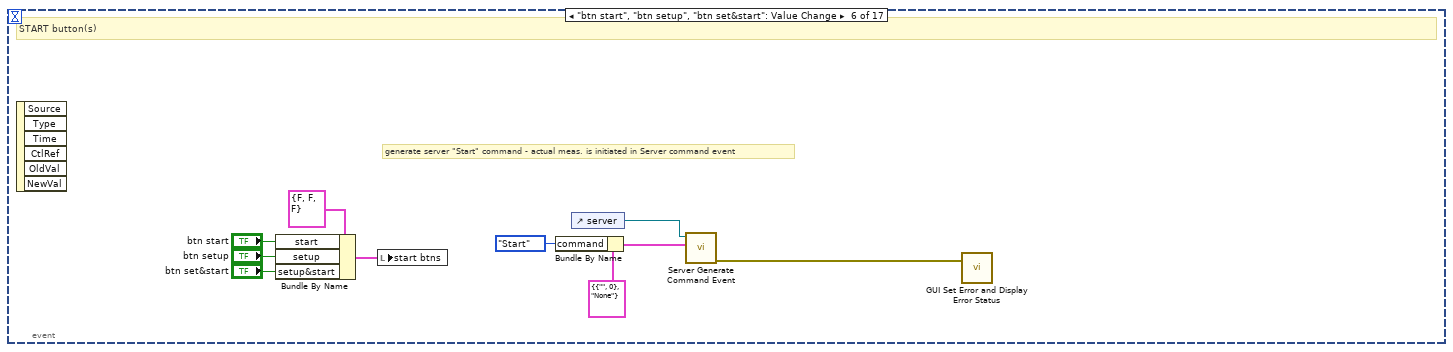
[diagram p15: hidden frame]
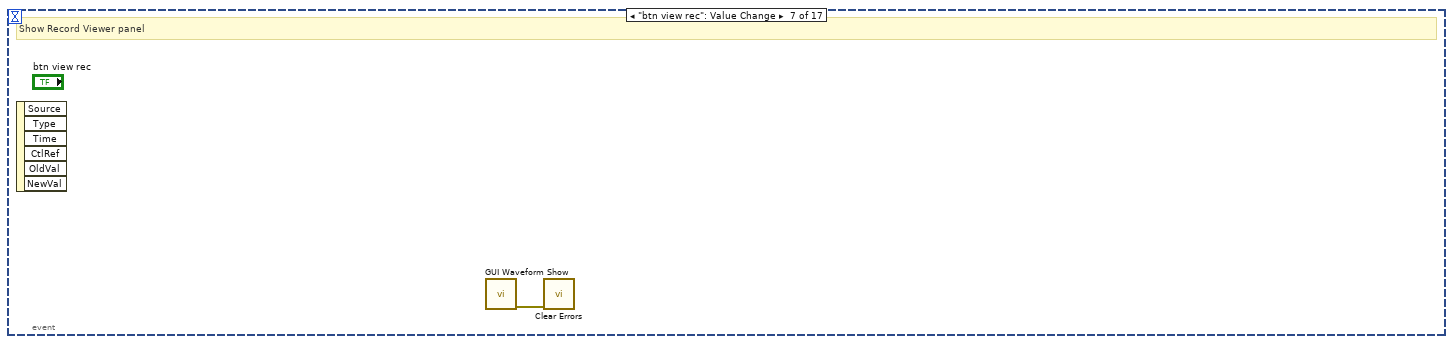
[diagram p16: hidden frame]
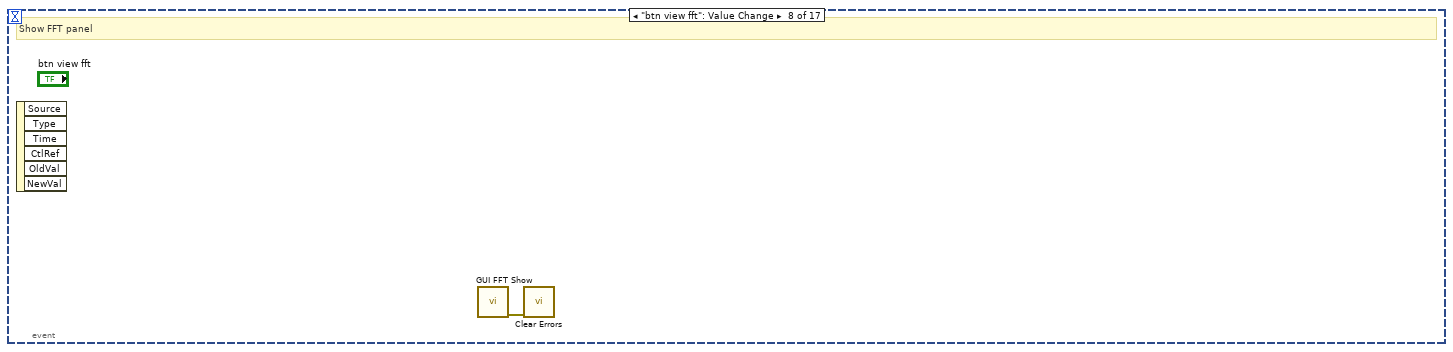
[diagram p17: hidden frame]
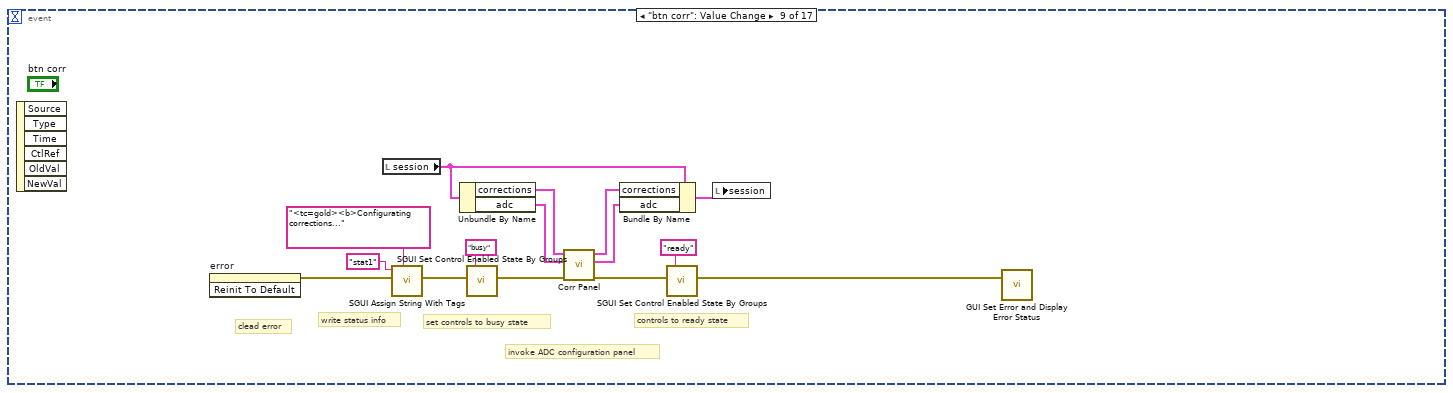
[diagram p18: hidden frame]
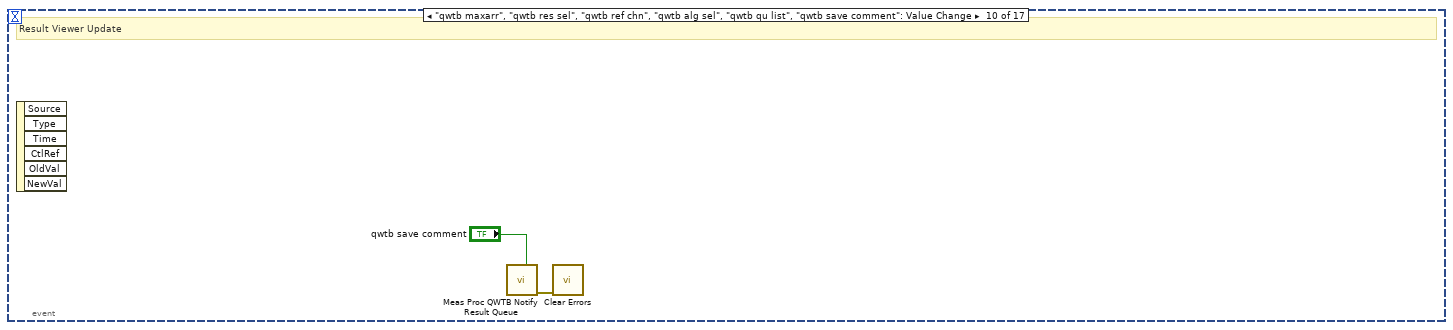
[diagram p19: hidden frame]
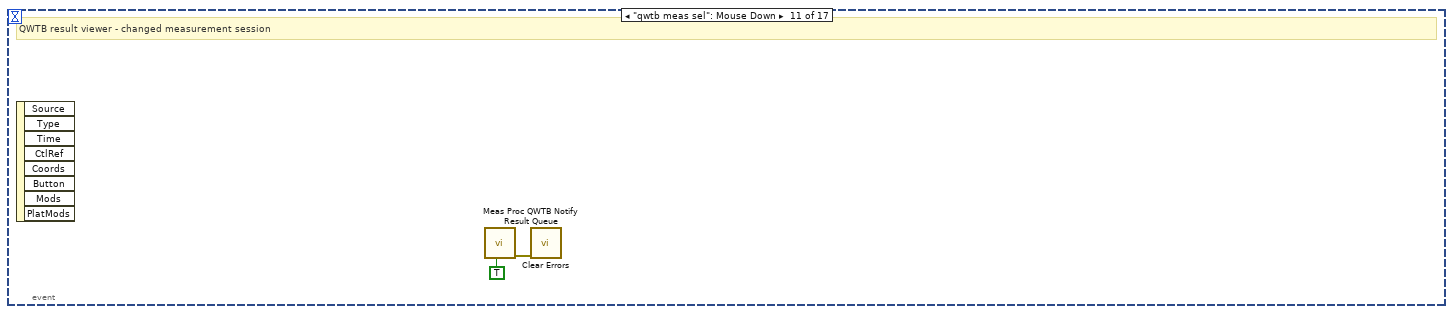
[diagram p20: hidden frame]
diagram:
  # "initialize GUI scaler"
  # "init FFT viewer"
  # "enable server button"
  # "init wave viewer"
  # "set controls to ready state"
  # "clear status lines"
  # "register front panel\nreference - this will\nbe used later to align\nsubpanels to main panel"
  # "restore session\nsetup from file"
  # "!!! local variables, no touchy !!!"
  # "clear stop\nbutton"
  # "synchronization"
  # "set controls to busy state"
  # "register control groups:\nby setting group state to\n'ready' or 'busy' all controls\nin the active group will go\nenabled, all others will go\ndisabled and grayed"
  # "register all controls on\nthe main VI panel for \nfurther access to them\nby their name (SGUI lib)"
  n1 = control-ref of="server"() -> (w18:refnum<vi>)
  n2 = vi-ref "main.vi"() -> (w3:refnum<vi>)
  n3 = vi-ref "Assist Sampling Measure Freq Panel.vi"() -> (w26:refnum<vi>)
  n4 = vi-ref "Meas Proc QWTB Result Plot Panel.vi"() -> (w24:refnum<vi>)
  n5 = vi-ref "Meas Proc QWTB Export Result.vi"() -> (w11:refnum<vi>)
  n6 = vi-ref "GUI FFT panel 2x.vi"() -> (w1:refnum<vi>)
  n7 = call "Scale Controls Helper.vi"("Action (Initialize)"=enum16{"Initialize", "Resize", "Resize?"}."Initialize", "vi reference"=w3) -> ("error out"=w4:errorcluster)  [unwired: 9 in]
  n8 = control-ref of="session"() -> (w41:refnum<vi>)
  n9 = control-ref of="golpi"() -> (w37:refnum<vi>)
  n10 = control-ref of="qwtb view"() -> (w28:refnum<vi>)
  n11 = call "Server Create Command Event.vi"("server ref"=w18) -> ("error out"=w20:errorcluster, "server command event"=w22:refnum<user-event>)  [unwired: 9 in]
  n12 = Build Array(w26, w24, w11, w1) -> (w25:refnum<vi>[])
  n13 = call "align_vi_panel.vi"("error in"=w4, "top vi reference"=w3) -> ("error out"=w40:errorcluster)  [unwired: 9 in]
  n14 = control-ref of="btn set&start"() -> (w29:refnum<vi>)
  n15 = control-ref of="btn start"() -> (w54:refnum<vi>)
  n16 = control-ref of="btn exit"() -> (w53:refnum<vi>)
  n17 = control-ref of="btn cfg octave"() -> (w52:refnum<vi>)
  n18 = control-ref of="btn cfg adc"() -> (w51:refnum<vi>)
  n19 = control-ref of="btn setup"() -> (w31:refnum<vi>)
  n20 = control-ref of="btn corr"() -> (w30:refnum<vi>)
  n21 = control-ref of="btn qwtb calc"() -> (w27:refnum<vi>)
  n22 = call "Server Create Response Event.vi"("error in"=w20, "server ref"=w18) -> ("error out"=w19:errorcluster)  [unwired: 8 in, 1 out]
  n23 = Build Array(w41, w37, w28) -> (w34:refnum<vi>[])
  n24 = control-ref of="btn stop"() -> (w48:refnum<vi>)
  n25 = register-events(w22) -> (reference out=w23:refnum<event-registration>)  [unwired: 2 in, 1 out]
  n26 = call <vilib>:"Clear Errors.vi"("error in (no error)"=w19) -> ()  [unwired: 5 in, 2 out]
  n27 = Build Array(w29, w54, w53, w52, w51, w31, w30, w27) -> (w55:refnum<vi>[])
  n28 = Build Array(w48) -> (w49:refnum<vi>[])
  n29 = call "SGUI Register Controls.vi"("error in"=w40, "register mode (overwrite)"=SGUI_Assign_References_Mode."Overwrite") -> ("error out"=w58:errorcluster)  [unwired: 15 in, 2 out]
  n30 = Bundle(w55) -> (w56:cluster{refnum<vi>[]})  [unwired: 1 in]
  n31 = Bundle(w49) -> (w50:cluster{refnum<vi>[]})  [unwired: 1 in]
  n32 = Build Array(w56, w50) -> (w57:cluster{refnum<vi>[]}[])
  n33 = call "SGUI Register Controls Groups.vi"("control groups"=w57, "error in"=w58, "groups names"="ready\nbusy", "register mode (overwrite)"=SGUI_Assign_References_Mode."Overwrite") -> ("error out"=w45:errorcluster)  [unwired: 14 in, 1 out]
  n34 = disable-structure shown="Disabled" {
    frame Disabled {
      # "programatic labeling of decorations, because LV GUI cannot do it!"
      n35 = property on="tc result" class="TabCtl (strict)"() -> (error out=w64:errorcluster, "Pages"=w62:refnum<vi>[])  [unwired: 2 in, 1 out]
      n36 = Index Array(array=w62) -> (element #2=w63:refnum<vi>)  [unwired: 2 in, 1 out]
      n37 = property class="Page"(reference=w63, error in=w64) -> ("DecosOnPage"=w61:refnum<vi>[])  [unwired: 2 out]
      n38 = for {
        tunnel: w61 -> [w66] mode=indexing
        tunnel: string[] ["qwtb res vert1 decor", "qwtb res horz decor"] -> [w65] mode=indexing
        n39 = call "Set Decoration Label.vi"("Label"=w65, "Decor Refnum"=w66) -> ()  [unwired: 4 in, 2 out]
      }
    }
    frame Enabled {
    }
  }
  n40 = call "SGUI Set Control Enabled State By Groups.vi"("error in"=w45, "group name to enable (none)"="busy") -> ("error out"=w17:errorcluster)  [unwired: 8 in, 1 out]
  n41 = call "SGUI Set Control Enabled State By Label.vi"("error in"=w17, "labels (empty)"="btn srv" ("control label(s) ('btn stop')"), "Enabled? (False)"=TRUE) -> ("error out"=w16:errorcluster)  [unwired: 7 in, 1 out]
  n42 = call-poly "SGUI Assign String With Tags.vi"("error in"=w16, "label(s) (empty)"="stat1\nstat2\nstat3\nstat4", "string (empty)"="<al=left><tc=gold><b>\n<al=left><tc=gold><b>\n<al=left><tc=gold><b>\n<al=left><tc=gold><b>") -> ("error out"=w36:errorcluster)  [unwired: 7 in, 1 out]
  n43 = call "SGUI Set Boolean State By Label.vi"("error in"=w36, "control label(s) ('btn stop')"="btn stop") -> ("error out"=w9:errorcluster)  [unwired: 8 in, 1 out]
  n44 = call "ini_load_variables.vi"("error in"=w9, "VI to store"=w25, "objects to store"=w34) -> ("error out"=w10:errorcluster, "config.ini not found?"=w6:bool)  [unwired: 7 in]
  n45 = call <vilib>:"Clear Errors.vi"("error in (no error)"=w10) -> ("error out"=w8:errorcluster)  [unwired: 5 in, 1 out]
  n46 = Merge Errors(w9, w8) -> (w7:errorcluster)
  n47 = flat-sequence {
    tunnel: w7 -> [w106]
    tunnel: [w73] -> w35
    tunnel: w6 -> [w70]
    frame #0 {
      # "local variable\nwith references\nto the QWTB result\nviewer"
      # "QWTB algorithms database, #todo: should be moved somwhere else"
      # "create QWTB result\nnotify queue"
      # "initialize GOLPI\nfor Octave calculations"
      # "new ADC HW set\nso set modified flag"
      # "initialize ADC drivers and otehr stuff"
      n48 = local read "session"() -> (w104:T13)
      n49 = Unbundle By Name(w104) -> ("processing setup"=w100:T100, "adc"=w105:T14)
      n50 = call "ADC Initialize Drivers.vi"("error in"=w106, "adc session in"=w105) -> ("error out"=w80:errorcluster, "adc session out"=w77:T14)  [unwired: 8 in]
      n51 = invoke on="qwtb results table" class="Tbl (strict)" method="Reinit To Default"() -> (error out=w69:errorcluster)  [unwired: 3 in, 2 out]
      n52 = control-ref of="golpi"() -> (w101:refnum<vi>)
      n53 = call "ADC Update and Check Idle Timer.vi"("error in"=w80, "adc session in"=w77) -> ("error out"=w79:errorcluster, "adc session out"=w78:T14)  [unwired: 6 in, 2 out]
      n54 = invoke on="qwtb qu list" class="LstBox (strict)" method="Reinit To Default"(error in=w69) -> (error out=w68:errorcluster)  [unwired: 2 in, 2 out]
      n55 = call "GOLPI Initialize.vi"("processing setup"=w100, "error in"=w79, "golpi session ref"=w101) -> ("error out"=w99:errorcluster, "golpi session out (copy)"=w102:T99)  [unwired: 6 in, 1 out]
      n56 = control-ref of="tc result"() -> (w83:refnum<vi>)
      n57 = control-ref of="qwtb qu list"() -> (w81:refnum<vi>)
      n58 = control-ref of="qwtb maxarr"() -> (w87:refnum<vi>)
      n59 = control-ref of="qwtb res info"() -> (w90:refnum<vi>)
      n60 = control-ref of="qwtb meas pth"() -> (w95:refnum<vi>)
      n61 = control-ref of="qwtb comment"() -> (w76:refnum<vi>)
      n62 = control-ref of="qwtb maxdim"() -> (w84:refnum<vi>)
      n63 = control-ref of="qwtb unc"() -> (w85:refnum<vi>)
      n64 = control-ref of="qwtb order"() -> (w86:refnum<vi>)
      n65 = control-ref of="qwtb results table"() -> (w89:refnum<vi>)
      n66 = control-ref of="qwtb ph unit"() -> (w92:refnum<vi>)
      n67 = control-ref of="qwtb amp"() -> (w67:refnum<vi>)
      n68 = control-ref of="qwtb res sel"() -> (w88:refnum<vi>)
      n69 = control-ref of="qwtb ref chn"() -> (w91:refnum<vi>)
      n70 = control-ref of="qwtb alg sel"() -> (w93:refnum<vi>)
      n71 = control-ref of="qwtb meas sel"() -> (w94:refnum<vi>)
      n72 = call <vilib>:"Clear Errors.vi"("error in (no error)"=w68) -> ()  [unwired: 5 in, 2 out]
      n73 = Bundle By Name(cluster=w104, "processing setup.QWTB.octave reset"=TRUE, "processing setup.QWTB.alg filter path"="octprog\\qwtb_list.info", "adc"=w78, "adc.modified?"=TRUE, "golpi"=w102) -> (w98:T13)
      n74 = local read "qwtb view"() -> (w82:T3)
      n75 = Bundle By Name(cluster=w82, "tc result"=w83, "qwtb maxdim"=w84, "qwtb unc"=w85, "qwtb order"=w86, "qwtb maxarr"=w87, "qwtb res sel"=w88, "qwtb results tbl"=w89, "qwtb res info"=w90, "qwtb ph unit"=w92, "qwtb ref chn"=w91, "qwtb alg sel"=w93, "qwtb meas sel"=w94, "qwtb ssn info"=w95, "qwtb qu list"=w81, "qwtb amp"=w67, "qwtb comment"=w76) -> (w96:T3)
      n76 = local write "qwtb view"(w96) -> ()
      n77 = call "Meas Proc QWTB Initialize Result Queue.vi"("error in"=w99, "session in"=w98) -> ("error out"=w74:errorcluster, "session out"=w72:T13)  [unwired: 8 in]
      n78 = case shown="True" w70 {
        tunnel: w74 -> [w108 w114]
        tunnel: [w108 w111] -> w73
        tunnel: w72 -> [w107 w113]
        tunnel: [w107 w110] -> w71
        frame False {
        }
        frame True {
          n79 = call "Meas Default.vi"("error in (no error)"=w114, "session in"=w113) -> ("error out"=w112:errorcluster, "session out"=w109:T13)  [unwired: 8 in]
          n80 = call "GOLPI Set Default Values.vi"("error in"=w112, "session in"=w109) -> ("error out"=w111:errorcluster, "session out"=w110:T13)  [unwired: 8 in]
        }
      }
      n81 = local write "session"(w71) -> ()
    }
  }
  n82 = flat-sequence {
    tunnel: w42 -> [_]
    tunnel: w34 -> [w128]
    tunnel: w25 -> [w124]
    tunnel: w21 -> [w123]
    frame #0 {
      w121 = TRUE ("Destroy notifier (False)")
      # "destroy QWTB result\nnotify queue"
      # "close GOLPI\nif was opened"
      # "store session\nsetup to file"
      # "controls ready"
      # "on exit event"
      n83 = Unregister For Events(event registration refnum=w123) -> (error out=w122:errorcluster)  [unwired: 1 in]
      n84 = call "SGUI Set Control Enabled State By Groups.vi"("error in"=w122, "group name to enable (none)"="ready") -> ("error out"=w120:errorcluster)  [unwired: 8 in, 1 out]
      n85 = call "GUI FFT Update.vi"("Destroy notifier (False)"=w121, "error in"=w120) -> ("error out"=w116:errorcluster)  [unwired: 9 in]
      n86 = call "GUI Waveform Update.vi"("Destroy notifier (False)"=w121, "error in"=w120) -> ("error out"=w117:errorcluster)  [unwired: 9 in]
      n87 = call "ini_save_variables.vi"("error in"=w120, "VI to store"=w124, "objects"=w128) -> ("error out"=w118:errorcluster)  [unwired: 8 in]
      n88 = Merge Errors(w116, w117, w118) -> (w115:errorcluster)
      n89 = control-ref of="golpi"() -> (w127:refnum<vi>)
      n90 = call "golpi_mpc_close_session.vi"("error in"=w115, "golpi session ref"=w127) -> ("error out"=w119:errorcluster)  [unwired: 8 in, 1 out]
      n91 = local read "session"() -> (w125:T13)
      n92 = call "Meas Proc QWTB Close Result Queue.vi"("error in"=w119, "session in"=w125) -> ("error out"=w126:errorcluster)  [unwired: 8 in, 1 out]
      n93 = call "GUI Set Error and Display Error Status.vi"("error in"=w126) -> ()  [unwired: 4 in]
    }
    frame #1 {
      # "last action - exit LV"
      n94 = call "Get Application Version.vi"() -> ("run time system"=w130:bool)  [unwired: 8 in, 3 out]
      n95 = Quit LabVIEW(quit? (T)=w130) -> ()
    }
  }
  n96 = call "GUI Waveform Update.vi"("error in"=w35) -> ("error out"=w13:errorcluster)  [unwired: 10 in]
  n97 = call "GUI FFT Update.vi"("error in"=w13) -> ("error out"=w12:errorcluster)  [unwired: 10 in]
  n98 = call "SGUI Set Control Enabled State By Groups.vi"("error in"=w12, "group name to enable (none)"="ready") -> ("error out"=w32:errorcluster)  [unwired: 8 in, 1 out]
  n99 = call "GUI Set Error and Display Error Status.vi"("error in"=w32) -> ()  [unwired: 4 in]
  n100 = call <vilib>:"Clear Errors.vi"("error in (no error)"=w32) -> ("error out"=w5:errorcluster)  [unwired: 5 in, 1 out]
  n101 = while {
    tunnel: w5 -> [_]
    tunnel: [w133] -> w42
    tunnel: w23 -> [w132]
    tunnel: [w131] -> w21
    stop <- w133 stop-if-true
    # "Main GUI Control Loop"
    n102 = event shown="[15] <server command event>: User Event" {
      selector: w132 -> [_ _ _ _ _ _ _ _ _ _ _ _ _ _ _ _ _]
      dyn-events: [_ _ _ _ _ _ _ _ _ _ _ _ _ _ _ _ _] -> w131
      timeout: 50 -> [_ _ _ _ _ _ _ _ _ _ _ _ _ _ _ _ _]
      tunnel: [_ TRUE _ _ _ _ _ _ _ _ _ _ _ _ _ _ _] -> w133
      event Timeout {
        # "GUI panel resizer"
        # "DELAYED DIGITIZER RESET CHECK"
        # "CHECK SERVER PANEL EXIT"
        # "RESULT VIEWER UPDATE"
        # "check measurement\nVI exit status"
        # "TIMER - periodic checks of everything"
        n103 = event-data() -> ()  [unwired: 1 in, 3 out]
        n104 = call "SGUI Get Boolean State By Label.vi"() -> ("error out"=w161:errorcluster, "binary state out"=w160:bool)  [unwired: 9 in, 1 out]
        n105 = local read "qwtb view VI ref"() -> (w153:refnum<vi>)
        n106 = case shown="True" w160 {
          tunnel: w161 -> [w195 w199]
          tunnel: [w195 w197] -> w159
          frame False {
          }
          frame True {
            # "gray stop when\npressed"
            n107 = call "SGUI Set Control Enabled State By Label.vi"("error in"=w199, "labels (empty)"="btn stop", "Enabled? (False)"=FALSE) -> ("error out"=w197:errorcluster)  [unwired: 7 in, 1 out]
          }
        }
        n108 = local read "qwtb view"() -> (w157:T3)
        n109 = local read "session"() -> (w158:T13)
        n110 = call "Meas Proc QWTB Update Result View.vi"("QWTB result session in"=w157, "async VI reference in"=w153, "session in"=w158) -> ("error out"=w156:errorcluster, "async VI reference out"=w154:refnum<vi>, "VI returned?"=w152:bool, "QWTB result session out"=w155:T3)  [unwired: 4 in, 1 out]
        n111 = local read "session VI ref"() -> (w162:refnum<vi>)
        n112 = case shown="True" w152 {
          tunnel: w155 -> [_ w194]
          frame False {
          }
          frame True {
            n113 = local write "qwtb view"(w194) -> ()
          }
        }
        n114 = call <vilib>:"Clear Errors.vi"("error in (no error)"=w156) -> ()  [unwired: 5 in, 2 out]
        n115 = local write "qwtb view VI ref"(w154) -> ()
        n116 = call "Meas Asynchronous Wait.vi"("Wait for exit? (False)"=FALSE, "error in"=w159, "VI reference (empty)"=w162) -> ("error out"=w165:errorcluster, "VI's error out"=w166:errorcluster, "VI returned?"=w167:bool, "parameter out"=w163:variant)  [unwired: 4 in, 1 out]
        n117 = local read "session"() -> (w140:T13)
        n118 = call <vilib>:"Clear Errors.vi"("error in (no error)"=w165) -> ()  [unwired: 5 in, 2 out]
        n119 = case shown="True" w167 {
          tunnel: w166 -> [_ w207]
          tunnel: w163 -> [_ w208]
          tunnel: [w200 w202] -> w139
          tunnel: w140 -> [w200 _]
          frame False {
          }
          frame True {
            # "controls to ready"
            # "Measurement VI returned - store its return data\nback to measurement session"
            n120 = Variant To Data(type=T13 {"adc"={"niScope"={"channel cfg"=[], "sessions"=[], "multi cards"=FALSE, "channels"=0, "type"=enum."n/a", "memory [B/chn]"=0, "ext. clock [Hz]"=0.0, "samples count"=0, "use streaming"=FALSE, "proc setup"={"packet size [smpl]"=0, "current timeout [s]"=0.0, "blk2blk timeout [s]"=0.0, "event time"=timestamp(0 s since 1904-01-01), "temp sampl T [s]"=0.0, "data queue"=refnum, "stop notifier"=refnum, "proc ref"=refnum}, "sample width [B]"=0, "ranges [V]"=[], "trigger setup"={"coupling"=1, "level [V]"=0.0, "slope"=0, "mode"=enum."Immediate", "pre-trigger [%]"=0.0}, "fs [Hz]"=0.0, "bitres [bit]"=0, "clock source"=enum."VAL_NO_SOURCE"}, "3458A"={"channels"=[], "sync unit"={"VISA"="", "type"=enum."Picotest U6200A"}, "awg unit"={"type"=enum."Agilent 331xxA to 332xxA", "VISA"="", "enable 10MHz ref"=FALSE, "cmi ckd2"={"VISA"="", "clock source"=enum."Auto", "manual ref clk"=FALSE, "ref clock [Hz]"=0.0, "div mode"=enum."Set divisor directly"}, "cmi sync v3"={"VISA"="", "baud rate [bd/s]"=115200, "source"=enum."Auto", "hv range"=enum."1kV", "fsrc is fixed"=FALSE, "fsrc [Hz]"=10000000.0, "freq integ [s]"=1.0, "freq filter"=5, "trig level"=enum."TTL 5V", "chn1 mode"=enum."Source divider", "chn1 level"=enum."Positive 5V", "chn2 mode"=enum."Source divider", "chn2 level"=enum."Positive 5V", "chn2 div"=1, "chn3 mode"=enum."Chn 1 Active", "chn3 level"=enum."Positive 5V", "chn1 div entry"=enum."Calculate nearest divisor from measured fx", "chn1 dev limit [%]"=1.0, "chn1 check dev"=FALSE}, "trigger"={"source"=enum."Immediate", "slope"=enum."POS", "coupling"=enum."DC", "level [V]"=0.0, "hysteresis [V]"=0.0, "pre-trigger [%]"=0.0}, "HMF2500 cfg"={"Baud Rate"=9600, "Parity"=0, "Data Bits"=8, "Flow Control"=4}}, "sync mode"=enum."MASTER-SLAVE, MASTER clocked by TIMER", "streaming mode"=FALSE, "idn mode"=enum."Auto", "sampling mode"=enum."DCV", "sample memory [B]"=0, "proc setup"={"channel id"=0, "packet size [smpl]"=0, "current timeout [s]"=0.0, "blk2blk timeout [s]"=0.0, "event time"=timestamp(0 s since 1904-01-01), "stop notifier"=refnum, "data queues"=[], "proc refs"=[], "bus semaphore"=refnum}, "sample size [B]"=0, "sample count"=0, "aux data"={"channel id"=0, "valid?"=[], "gain [V]"=[], "timestamp [s]"=[], "Ts [s]"=0.0, "abs timestamp"=timestamp(0 s since 1904-01-01), "t [deg C]"=[], "multiplex timestamp [s]"=-1.0, "only multiplex?"=FALSE, "multiplex smpl offset"=0, "overflow?"=FALSE}, "ranges [V]"=[], "aperture [s]"=0.0, "LEVEL trigger"={"edge"=enum."POS", "level [V]"=0.0, "coupling"=enum."DC"}, "trigger mode"=enum."AUTO", "measure temp.?"=FALSE, "disp mesages"=[], "shared bus?"=FALSE, "disable display?"=FALSE, "aper mode"=enum."Manual", "aper rules"=[], "multiplex"={"cycles"=0, "delay [s]"=0.0, "enabled"=FALSE, "overhead [s]"=1.0, "tot smpls"=0, "sub-rec"=0, "overhead [%]"=0.0, "emulated"=FALSE}, "F8588 lpf"=enum."Off", "F8588 pll"=enum."Off", "F8588 couple"=enum."DC, auto", "fs"={"freq mode"=enum."fs or Ts", "fs [Hz]"=0.0, "fref [Hz]"=0.0, "mul"=0.0, "div"=0.0}, "fs mode"=enum."fs or Ts"}, "dsdll"={"dsdll"={"dsdll path"=path "", "dsdll handle"=[], "output devices"=[], "capture devices"=[]}, "channels"=0, "device id"=0, "channel idns"=[], "proc setup"={"packet size [smpl]"=0, "current timeout [s]"=0.0, "blk2blk timeout [s]"=0.0, "event time"=timestamp(0 s since 1904-01-01), "data queue"=refnum, "stop notifier"=refnum, "proc ref"=refnum}, "samples count"=0, "fs [Hz]"=0.0}, "type"=enum."niScope", "channel idn str"=[], "aux instr idn str"=[], "modified?"=FALSE, "simadc"={"channels"=[], "range [V]"=0.0, "Ts step [s]"=0.0, "time [s]"=0.0, "fs [Hz]"=0.0, "count"=0, "smpl offset"=0, "set count"=0, "bit res"=0}, "force rst?"=FALSE, "exit mode"=enum."Immediate reset", "exit dly"=0.0, "exit tmr"=timestamp(0 s since 1904-01-01), "busy?"=FALSE, "accessed?"=FALSE, "multiplex"={"Type"=enum."Dummy", "gen com ssn"={"visa"="", "primary"=enum."None", "secondary"=enum."None", "channels"=[]}, "delay before [s]"=0.0, "delay post [s]"=0.0, "sequence"=[], "enabled"=FALSE, "ref timestamp [s]"=0.0, "idn string"="", "dev niScope"="", "niScope idx"=0, "QPMX ssn"={"visa"="", "switch mode"=enum."Switched by TWM", "sequence"=[], "timing delays"=[], "polarity"=enum."Positive", "ss delay (s)"=2.0, "internal timer (s)"=1.0, "Last loaded sequence file"=path "", "startup delay (s)"=2.0}, "VISA mux ssn"={"VISA"="", "paths"=[], "idn command"="", "serial cfg"={"Baud rate"=9600, "Data bits"=8, "Parity"=0, "Stop bits"=10, "Flow control"=0, "End Mode Read"=enum."None", "End Mode Write"=enum."None", "Term character"=0, "Term enable"=FALSE}}}, "keysight dso"={"VISA"="", "channels"=[], "bw limit [Hz]"=0.0, "resolution"=enum."Basic", "trig noise reject"=enum."Normal", "N"=0, "trigger config"={"trigger source"=enum."Immediate", "trigger slope"=enum."Negative", "level [V]"=0.0, "hysteresis [V]"=0.001, "pre-trig [%]"=50}, "fs [Hz]"=0.0, "timeout stop"=timestamp(0 s since 1904-01-01), "waiting for opc"=FALSE, "fetch offset [smpl]"=0, "abs timestamp"=timestamp(0 s since 1904-01-01), "ranges [V]"=[], "decimation"=1.0, "ext ref"=FALSE, "emulate aperture"=FALSE, "model"=enum."DSO91304"}, "cdaq"={"mclk [Hz]"=12800000.0, "ADC task"="", "mclk reference"="", "fs [Hz]"=50000.0, "queue adc cmd"=refnum, "queue adc data"=refnum, "adc proc ref"=refnum, "channels"=[], "last channels"=[], "timeout"=timestamp(0 s since 1904-01-01), "N"=1000, "mclk mode"=enum."Free running", "ext mclk source"=""}, "ignore overload"=FALSE}, "sequence"=[], "sequence setup"={"group setups"=[], "rec count"=0, "range mode"=enum."Keep defaults", "fs mode"=enum."Frequency", "rng even"=0.0, "rng odd"=0.0, "folder"=path "", "name base"="", "meas id"=0, "settle [s]"=0.0, "comment"="", "avg count"=0, "fs-abs-fr fr"=0.0, "fs-abs-fr fs"=0.0, "fs-div fr"=0.0, "fs-div div"=0.0, "fs-mn fr"=0.0, "fs-mn mul"=0.0, "fs-mn div"=0.0, "fs-rat fr"=0.0, "fs-rat rat"=0.0}, "golpi"=refnum, "processing setup"={"mode"=enum."Raw", "call after avgs?"=FALSE, "calculate?"=FALSE, "raw mode"={"command"="", "result mode"=enum."Display console output (only Octave)", "res variable"=""}, "QWTB"={"QWTB path"=path "", "alg filter path"="", "alg ids"=[], "alg parameters"=[], "parsed parameters"=[], "selected alg id"="", "selected unc mode"=enum."None", "qwtb mcc"=100, "qwtb timeout"=90, "qwtb covg"=95.0, "qwtb ofs"=0, "qwtb lim data"=0, "multicore"={"jobs folder"=path "", "cores"=0, "max jobs"=0, "mode"=enum."Singlecore"}, "unc once?"=FALSE, "qwtb tstemp"=enum."Enabled (default)", "octave reset"=FALSE, "exec mode"=enum."Single-core"}}, "corrections"={"transducers"={"channels"=[], "last path"=path "", "root path"=path ""}, "digitizer"={"last path"=path "", "channel paths"=[], "channel idns"=[], "correction name"="", "channel names"=[], "folders to copy"=[], "channel valid"=[], "correction path"=path "", "correction rel path"="", "rel folders to copy"=[], "root path"=path ""}}, "assist cfg"={"P"=0, "Q"=0, "rel shift"=0.0, "ref freq"=0.0, "min fs"=0.0, "max fs tol"=0.0, "min int"=0.0, "max int"=0.0, "max err"=0.0, "max timeout"=0.0}} ("session"), Variant=w208) -> (data=w202:T13, error out=w206:errorcluster)  [unwired: 1 in]
            n121 = Merge Errors(w207, w206) -> (w205:errorcluster)
            n122 = call "SGUI Set Control Enabled State By Groups.vi"("error in"=w205, "group name to enable (none)"="ready") -> ("error out"=w204:errorcluster)  [unwired: 8 in, 1 out]
            n123 = call "GUI Set Error and Display Error Status.vi"("error in"=w204) -> ()  [unwired: 4 in]
          }
        }
        n124 = vi-ref "main.vi"() -> (w138:refnum<vi>)
        n125 = call "Scale Controls Helper.vi"("rules"="tc result [edge:LRTB]\nbtn view rec [edge:R]\nbtn view fft [edge:R]\nbtn srv [edge:R]\nbtn about [edge:R]\nstat1 [edge:LR]\nstat2 [edge:LR]\nstat3 [edge:LR]\nstat4 [edge:LR]\nbtn exit [edge:RB]\nerror [edge:B]\nqwtb results table [edge:LRTB]\nqwtb qu list [edge:TBR]\nqwtb res info [edge:LR]\nqwtb comment [edge:LR]\nqwtb save comment [edge:R]\nqwtb alg sel [edge:LR]\nqwtb res horz decor [edge:LR]\nstr res [edge:LRTB]", "Action (Initialize)"=enum16{"Initialize", "Resize", "Resize?"}."Resize?", "vi reference"=w138) -> ("error out"=w135:errorcluster)  [unwired: 8 in]
        n126 = call <vilib>:"Clear Errors.vi"("error in (no error)"=w135) -> ()  [unwired: 5 in, 2 out]
        n127 = Unbundle By Name(w139) -> ("adc"=w147:T14)
        n128 = call "ADC Update and Check Idle Timer.vi"("adc session in"=w147) -> ("error out"=w145:errorcluster, "timeout?"=w144:bool, "adc session out"=w146:T14)  [unwired: 7 in, 1 out]
        n129 = local read "server vi ref"() -> (w151:refnum<vi>)
        n130 = case shown="True" w144 {
          tunnel: w146 -> [w168 w187]
          tunnel: w145 -> [w169 w180]
          tunnel: [w168 w184] -> w142
          tunnel: [w169 w170] -> w143
          frame False {
          }
          frame True {
            # "FORCE RESET"
            n131 = call "SGUI Set Control Enabled State By Groups.vi"("error in"=w180, "group name to enable (none)"="busy") -> ("error out"=w177:errorcluster)  [unwired: 8 in, 1 out]
            n132 = call-poly "SGUI Assign String With Tags.vi"("error in"=w177, "label(s) (empty)"="stat2", "string (empty)"="<tc=gold><b>Reseting digitizer to idle...") -> ("error out"=w176:errorcluster)  [unwired: 7 in, 1 out]
            n133 = call "ADC Initialize Virtual Channels.vi"("error in"=w176, "Reset? (False)"=FALSE, "adc session in"=w187) -> ("error out"=w189:errorcluster, "adc session out"=w188:T14)  [unwired: 3 in, 4 out]
            n134 = call "ADC Close Virtual Channels.vi"("error in"=w189, "Force reset to preset mode (False)"=TRUE, "adc session in"=w188) -> ("error out"=w178:errorcluster, "adc session out"=w183:T14)  [unwired: 7 in]
            n135 = Bundle By Name(cluster=w183, "accessed?"=FALSE) -> (w184:T14)
            n136 = call "SGUI Set Control Enabled State By Groups.vi"("error in"=w178, "group name to enable (none)"="ready") -> ("error out"=w171:errorcluster)  [unwired: 8 in, 1 out]
            n137 = call-poly "SGUI Assign String With Tags.vi"("error in"=w171, "label(s) (empty)"="stat2", "string (empty)"="<tc=gold><b>Digitizer was set to idle.") -> ("error out"=w170:errorcluster)  [unwired: 7 in, 1 out]
          }
        }
        n138 = call "Meas Asynchronous Wait.vi"("VI reference (empty)"=w151) -> ("error out"=w148:errorcluster, "VI's error out"=w149:errorcluster, "VI returned?"=w150:bool)  [unwired: 6 in, 2 out]
        n139 = case shown="True" w150 {
          tunnel: w149 -> [_ w193]
          frame False {
          }
          frame True {
            n140 = call "SGUI Set Control Enabled State By Label.vi"("error in"=w193, "labels (empty)"="btn srv", "Enabled? (False)"=TRUE) -> ("error out"=w190:errorcluster)  [unwired: 7 in, 1 out]
            n141 = call <vilib>:"Clear Errors.vi"("error in (no error)"=w190) -> ()  [unwired: 5 in, 2 out]
          }
        }
        n142 = call <vilib>:"Clear Errors.vi"("error in (no error)"=w148) -> ()  [unwired: 5 in, 2 out]
        n143 = Bundle By Name(cluster=w139, "adc"=w142) -> (w141:T13)
        n144 = call <vilib>:"Clear Errors.vi"("error in (no error)"=w143) -> ()  [unwired: 5 in, 2 out]
        n145 = local write "session"(w141) -> ()
      }
      event "btn exit": Value Change; Panel Close {
        # "CHECK SERVER PANEL EXIT"
        # "terminate QWTB results viewer process"
        # "force measurement\nVI to exit"
        # "EXIT application"
        n146 = event-data() -> ()  [unwired: 1 in, 3 out]
        n147 = local read "session VI ref"() -> (w222:refnum<vi>)
        n148 = local read "qwtb view VI ref"() -> (w217:refnum<vi>)
        n149 = call "Meas Asynchronous Wait.vi"("Wait for exit? (False)"=TRUE, "VI reference (empty)"=w222) -> ("error out"=w225:errorcluster, "VI's error out"=w226:errorcluster, "VI returned?"=w227:bool, "parameter out"=w223:variant)  [unwired: 5 in, 1 out]
        n150 = call "Meas Asynchronous Wait.vi"("Wait for exit? (False)"=TRUE, "VI reference (empty)"=w217) -> ("error out"=w219:errorcluster, "VI's error out"=w220:errorcluster)  [unwired: 5 in, 3 out]
        n151 = call <vilib>:"Clear Errors.vi"("error in (no error)"=w225) -> ()  [unwired: 5 in, 2 out]
        n152 = Merge Errors(w220, w219) -> (w218:errorcluster)
        n153 = case shown="True" w227 {
          tunnel: w226 -> [_ w235]
          tunnel: w223 -> [_ w236]
          frame False {
          }
          frame True {
            # "controls to ready"
            # "Measurement VI returned - store its return data\nback to measurement session"
            n154 = Variant To Data(type=T13 {"adc"={"niScope"={"channel cfg"=[], "sessions"=[], "multi cards"=FALSE, "channels"=0, "type"=enum."n/a", "memory [B/chn]"=0, "ext. clock [Hz]"=0.0, "samples count"=0, "use streaming"=FALSE, "proc setup"={"packet size [smpl]"=0, "current timeout [s]"=0.0, "blk2blk timeout [s]"=0.0, "event time"=timestamp(0 s since 1904-01-01), "temp sampl T [s]"=0.0, "data queue"=refnum, "stop notifier"=refnum, "proc ref"=refnum}, "sample width [B]"=0, "ranges [V]"=[], "trigger setup"={"coupling"=1, "level [V]"=0.0, "slope"=0, "mode"=enum."Immediate", "pre-trigger [%]"=0.0}, "fs [Hz]"=0.0, "bitres [bit]"=0, "clock source"=enum."VAL_NO_SOURCE"}, "3458A"={"channels"=[], "sync unit"={"VISA"="", "type"=enum."Picotest U6200A"}, "awg unit"={"type"=enum."Agilent 331xxA to 332xxA", "VISA"="", "enable 10MHz ref"=FALSE, "cmi ckd2"={"VISA"="", "clock source"=enum."Auto", "manual ref clk"=FALSE, "ref clock [Hz]"=0.0, "div mode"=enum."Set divisor directly"}, "cmi sync v3"={"VISA"="", "baud rate [bd/s]"=115200, "source"=enum."Auto", "hv range"=enum."1kV", "fsrc is fixed"=FALSE, "fsrc [Hz]"=10000000.0, "freq integ [s]"=1.0, "freq filter"=5, "trig level"=enum."TTL 5V", "chn1 mode"=enum."Source divider", "chn1 level"=enum."Positive 5V", "chn2 mode"=enum."Source divider", "chn2 level"=enum."Positive 5V", "chn2 div"=1, "chn3 mode"=enum."Chn 1 Active", "chn3 level"=enum."Positive 5V", "chn1 div entry"=enum."Calculate nearest divisor from measured fx", "chn1 dev limit [%]"=1.0, "chn1 check dev"=FALSE}, "trigger"={"source"=enum."Immediate", "slope"=enum."POS", "coupling"=enum."DC", "level [V]"=0.0, "hysteresis [V]"=0.0, "pre-trigger [%]"=0.0}, "HMF2500 cfg"={"Baud Rate"=9600, "Parity"=0, "Data Bits"=8, "Flow Control"=4}}, "sync mode"=enum."MASTER-SLAVE, MASTER clocked by TIMER", "streaming mode"=FALSE, "idn mode"=enum."Auto", "sampling mode"=enum."DCV", "sample memory [B]"=0, "proc setup"={"channel id"=0, "packet size [smpl]"=0, "current timeout [s]"=0.0, "blk2blk timeout [s]"=0.0, "event time"=timestamp(0 s since 1904-01-01), "stop notifier"=refnum, "data queues"=[], "proc refs"=[], "bus semaphore"=refnum}, "sample size [B]"=0, "sample count"=0, "aux data"={"channel id"=0, "valid?"=[], "gain [V]"=[], "timestamp [s]"=[], "Ts [s]"=0.0, "abs timestamp"=timestamp(0 s since 1904-01-01), "t [deg C]"=[], "multiplex timestamp [s]"=-1.0, "only multiplex?"=FALSE, "multiplex smpl offset"=0, "overflow?"=FALSE}, "ranges [V]"=[], "aperture [s]"=0.0, "LEVEL trigger"={"edge"=enum."POS", "level [V]"=0.0, "coupling"=enum."DC"}, "trigger mode"=enum."AUTO", "measure temp.?"=FALSE, "disp mesages"=[], "shared bus?"=FALSE, "disable display?"=FALSE, "aper mode"=enum."Manual", "aper rules"=[], "multiplex"={"cycles"=0, "delay [s]"=0.0, "enabled"=FALSE, "overhead [s]"=1.0, "tot smpls"=0, "sub-rec"=0, "overhead [%]"=0.0, "emulated"=FALSE}, "F8588 lpf"=enum."Off", "F8588 pll"=enum."Off", "F8588 couple"=enum."DC, auto", "fs"={"freq mode"=enum."fs or Ts", "fs [Hz]"=0.0, "fref [Hz]"=0.0, "mul"=0.0, "div"=0.0}, "fs mode"=enum."fs or Ts"}, "dsdll"={"dsdll"={"dsdll path"=path "", "dsdll handle"=[], "output devices"=[], "capture devices"=[]}, "channels"=0, "device id"=0, "channel idns"=[], "proc setup"={"packet size [smpl]"=0, "current timeout [s]"=0.0, "blk2blk timeout [s]"=0.0, "event time"=timestamp(0 s since 1904-01-01), "data queue"=refnum, "stop notifier"=refnum, "proc ref"=refnum}, "samples count"=0, "fs [Hz]"=0.0}, "type"=enum."niScope", "channel idn str"=[], "aux instr idn str"=[], "modified?"=FALSE, "simadc"={"channels"=[], "range [V]"=0.0, "Ts step [s]"=0.0, "time [s]"=0.0, "fs [Hz]"=0.0, "count"=0, "smpl offset"=0, "set count"=0, "bit res"=0}, "force rst?"=FALSE, "exit mode"=enum."Immediate reset", "exit dly"=0.0, "exit tmr"=timestamp(0 s since 1904-01-01), "busy?"=FALSE, "accessed?"=FALSE, "multiplex"={"Type"=enum."Dummy", "gen com ssn"={"visa"="", "primary"=enum."None", "secondary"=enum."None", "channels"=[]}, "delay before [s]"=0.0, "delay post [s]"=0.0, "sequence"=[], "enabled"=FALSE, "ref timestamp [s]"=0.0, "idn string"="", "dev niScope"="", "niScope idx"=0, "QPMX ssn"={"visa"="", "switch mode"=enum."Switched by TWM", "sequence"=[], "timing delays"=[], "polarity"=enum."Positive", "ss delay (s)"=2.0, "internal timer (s)"=1.0, "Last loaded sequence file"=path "", "startup delay (s)"=2.0}, "VISA mux ssn"={"VISA"="", "paths"=[], "idn command"="", "serial cfg"={"Baud rate"=9600, "Data bits"=8, "Parity"=0, "Stop bits"=10, "Flow control"=0, "End Mode Read"=enum."None", "End Mode Write"=enum."None", "Term character"=0, "Term enable"=FALSE}}}, "keysight dso"={"VISA"="", "channels"=[], "bw limit [Hz]"=0.0, "resolution"=enum."Basic", "trig noise reject"=enum."Normal", "N"=0, "trigger config"={"trigger source"=enum."Immediate", "trigger slope"=enum."Negative", "level [V]"=0.0, "hysteresis [V]"=0.001, "pre-trig [%]"=50}, "fs [Hz]"=0.0, "timeout stop"=timestamp(0 s since 1904-01-01), "waiting for opc"=FALSE, "fetch offset [smpl]"=0, "abs timestamp"=timestamp(0 s since 1904-01-01), "ranges [V]"=[], "decimation"=1.0, "ext ref"=FALSE, "emulate aperture"=FALSE, "model"=enum."DSO91304"}, "cdaq"={"mclk [Hz]"=12800000.0, "ADC task"="", "mclk reference"="", "fs [Hz]"=50000.0, "queue adc cmd"=refnum, "queue adc data"=refnum, "adc proc ref"=refnum, "channels"=[], "last channels"=[], "timeout"=timestamp(0 s since 1904-01-01), "N"=1000, "mclk mode"=enum."Free running", "ext mclk source"=""}, "ignore overload"=FALSE}, "sequence"=[], "sequence setup"={"group setups"=[], "rec count"=0, "range mode"=enum."Keep defaults", "fs mode"=enum."Frequency", "rng even"=0.0, "rng odd"=0.0, "folder"=path "", "name base"="", "meas id"=0, "settle [s]"=0.0, "comment"="", "avg count"=0, "fs-abs-fr fr"=0.0, "fs-abs-fr fs"=0.0, "fs-div fr"=0.0, "fs-div div"=0.0, "fs-mn fr"=0.0, "fs-mn mul"=0.0, "fs-mn div"=0.0, "fs-rat fr"=0.0, "fs-rat rat"=0.0}, "golpi"=refnum, "processing setup"={"mode"=enum."Raw", "call after avgs?"=FALSE, "calculate?"=FALSE, "raw mode"={"command"="", "result mode"=enum."Display console output (only Octave)", "res variable"=""}, "QWTB"={"QWTB path"=path "", "alg filter path"="", "alg ids"=[], "alg parameters"=[], "parsed parameters"=[], "selected alg id"="", "selected unc mode"=enum."None", "qwtb mcc"=100, "qwtb timeout"=90, "qwtb covg"=95.0, "qwtb ofs"=0, "qwtb lim data"=0, "multicore"={"jobs folder"=path "", "cores"=0, "max jobs"=0, "mode"=enum."Singlecore"}, "unc once?"=FALSE, "qwtb tstemp"=enum."Enabled (default)", "octave reset"=FALSE, "exec mode"=enum."Single-core"}}, "corrections"={"transducers"={"channels"=[], "last path"=path "", "root path"=path ""}, "digitizer"={"last path"=path "", "channel paths"=[], "channel idns"=[], "correction name"="", "channel names"=[], "folders to copy"=[], "channel valid"=[], "correction path"=path "", "correction rel path"="", "rel folders to copy"=[], "root path"=path ""}}, "assist cfg"={"P"=0, "Q"=0, "rel shift"=0.0, "ref freq"=0.0, "min fs"=0.0, "max fs tol"=0.0, "min int"=0.0, "max int"=0.0, "max err"=0.0, "max timeout"=0.0}} ("session"), Variant=w236) -> (data=w233:T13, error out=w234:errorcluster)  [unwired: 1 in]
            n155 = local write "session"(w233) -> ()
            n156 = Merge Errors(w235, w234) -> (w232:errorcluster)
            n157 = call "SGUI Set Control Enabled State By Groups.vi"("error in"=w232, "group name to enable (none)"="ready") -> ("error out"=w231:errorcluster)  [unwired: 8 in, 1 out]
            n158 = call "GUI Set Error and Display Error Status.vi"("error in"=w231) -> ()  [unwired: 4 in]
          }
        }
        n159 = call <vilib>:"Clear Errors.vi"("error in (no error)"=w218) -> ()  [unwired: 5 in, 2 out]
        n160 = local read "server vi ref"() -> (w216:refnum<vi>)
        n161 = call "Meas Asynchronous Wait.vi"("Wait for exit? (False)"=TRUE, "stop button name ('btn stop')"="btn srv exit", "VI reference (empty)"=w216) -> ("error out"=w214:errorcluster, "VI's error out"=w215:errorcluster)  [unwired: 4 in, 3 out]
        n162 = call <vilib>:"Clear Errors.vi"("error in (no error)"=w214) -> ()  [unwired: 5 in, 2 out]
        n163 = call "SGUI Set Control Enabled State By Label.vi"("error in"=w215, "labels (empty)"="btn srv", "Enabled? (False)"=TRUE) -> ("error out"=w209:errorcluster)  [unwired: 7 in, 1 out]
        n164 = call <vilib>:"Clear Errors.vi"("error in (no error)"=w209) -> ()  [unwired: 5 in, 2 out]
      }
      event "btn about": Value Change {
        # "show About dialog"
        n165 = event-data() -> ()  [unwired: 1 in, 6 out]
        n166 = call "About Dialog.vi"() -> ()  [unwired: 12 in]
      }
      event "btn cfg adc": Value Change {
        # "controls to ready state"
        # "clead error"
        # "write status info"
        # "set controls to busy state"
        # "invoke ADC configuration panel"
        # "Digitizer Configuration Panel"
        n167 = event-data() -> ()  [unwired: 1 in, 6 out]
        n168 = invoke on="error" class="Clust (strict)" method="Reinit To Default"() -> (error out=w241:errorcluster)  [unwired: 3 in, 2 out]
        n169 = call-poly "SGUI Assign String With Tags.vi"("error in"=w241, "label(s) (empty)"="stat1" ("control label (none)"), "string (empty)"="<tc=gold><b>Configurating Digitizer...") -> ("error out"=w240:errorcluster)  [unwired: 7 in, 1 out]
        n170 = local read "session"() -> (w248:T13)
        n171 = call "SGUI Set Control Enabled State By Groups.vi"("error in"=w240, "group name to enable (none)"="busy") -> ("error out"=w244:errorcluster)  [unwired: 8 in, 1 out]
        n172 = Unbundle By Name(w248) -> ("adc"=w249:T14)
        n173 = call "ADC Config Panel.vi"("error in"=w244, "adc session in"=w249) -> ("error out"=w242:errorcluster, "adc session out"=w247:T14)  [unwired: 8 in]
        n174 = Bundle By Name(cluster=w248, "adc"=w247) -> (w246:T13)
        n175 = local write "session"(w246) -> ()
        n176 = call "SGUI Set Control Enabled State By Groups.vi"("error in"=w242, "group name to enable (none)"="ready") -> ("error out"=w237:errorcluster)  [unwired: 8 in, 1 out]
        n177 = call "GUI Set Error and Display Error Status.vi"("error in"=w237) -> ()  [unwired: 4 in]
      }
      event "btn cfg octave": Value Change {
        # "controls to\nready state"
        # "clead error"
        # "write status info"
        # "set controls\nto busy state"
        # "Invoke GOLPI\nconfig panel"
        # "Digitizer Configuration Panel"
        n178 = event-data() -> ()  [unwired: 1 in, 6 out]
        n179 = invoke on="error" class="Clust (strict)" method="Reinit To Default"() -> (error out=w258:errorcluster)  [unwired: 3 in, 2 out]
        n180 = call-poly "SGUI Assign String With Tags.vi"("error in"=w258, "label(s) (empty)"="stat1" ("control label (none)"), "string (empty)"="<tc=gold><b>Configurating GOLPI interface...") -> ("error out"=w257:errorcluster)  [unwired: 7 in, 1 out]
        n181 = call "SGUI Set Control Enabled State By Groups.vi"("error in"=w257, "group name to enable (none)"="busy") -> ("error out"=w253:errorcluster)  [unwired: 8 in, 1 out]
        n182 = local read "session"() -> (w251:T13)
        n183 = call "GOLPI Config Panel.vi"("error in"=w253, "session in"=w251) -> ("error out"=w252:errorcluster, "session out"=w250:T13)  [unwired: 8 in]
        n184 = local write "session"(w250) -> ()
        n185 = call "SGUI Set Control Enabled State By Groups.vi"("error in"=w252, "group name to enable (none)"="ready") -> ("error out"=w254:errorcluster)  [unwired: 8 in, 1 out]
        n186 = call "GUI Set Error and Display Error Status.vi"("error in"=w254) -> ()  [unwired: 4 in]
      }
      event "btn start", "btn setup", "btn set&start": Value Change {
        # "generate server \"Start\" command - actual meas. is initiated in Server command event"
        # "START button(s)"
        n187 = event-data() -> ()  [unwired: 1 in, 6 out]
        n188 = Bundle By Name(cluster=T2 {"start"=FALSE, "setup"=FALSE, "setup&start"=FALSE} ("GUI request"), "start"="btn start", "setup"="btn setup", "setup&start"="btn set&start") -> (w262:T2)
        n189 = local write "start btns"(w262) -> ()
        n190 = Bundle By Name(cluster=T116 {"client request"={"info data"="", "answer handle"=0}, "command"=enum."None"} ("event data"), "command"=Server_Event_Command."Start") -> (w265:T116)
        n191 = control-ref of="server"() -> (w261:refnum<vi>)
        n192 = call "Server Generate Command Event.vi"("event data"=w265, "server event ref"=w261) -> ("error out"=w263:errorcluster)  [unwired: 9 in]
        n193 = call "GUI Set Error and Display Error Status.vi"("error in"=w263) -> ()  [unwired: 4 in]
      }
      event "btn view rec": Value Change {
        # "Show Record Viewer panel"
        n194 = event-data() -> ()  [unwired: 1 in, 6 out]
        n195 = call "GUI Waveform Show.vi"() -> ("error out"=w271:errorcluster)  [unwired: 11 in]
        n196 = call <vilib>:"Clear Errors.vi"("error in (no error)"=w271) -> ()  [unwired: 5 in, 2 out]
      }
      event "btn view fft": Value Change {
        # "Show FFT panel"
        n197 = event-data() -> ()  [unwired: 1 in, 6 out]
        n198 = call "GUI FFT Show.vi"() -> ("error out"=w272:errorcluster)  [unwired: 11 in]
        n199 = call <vilib>:"Clear Errors.vi"("error in (no error)"=w272) -> ()  [unwired: 5 in, 2 out]
      }
      event "btn corr": Value Change {
        # "controls to ready state"
        # "clead error"
        # "write status info"
        # "set controls to busy state"
        # "invoke ADC configuration panel"
        n200 = event-data() -> ()  [unwired: 1 in, 6 out]
        n201 = invoke on="error" class="Clust (strict)" method="Reinit To Default"() -> (error out=w281:errorcluster)  [unwired: 3 in, 2 out]
        n202 = local read "session"() -> (w287:T13)
        n203 = call-poly "SGUI Assign String With Tags.vi"("error in"=w281, "label(s) (empty)"="stat1" ("control label (none)"), "string (empty)"="<tc=gold><b>Configurating corrections...") -> ("error out"=w280:errorcluster)  [unwired: 7 in, 1 out]
        n204 = Unbundle By Name(w287) -> ("corrections"=w276:T110, "adc"=w274:T14)
        n205 = call "SGUI Set Control Enabled State By Groups.vi"("error in"=w280, "group name to enable (none)"="busy") -> ("error out"=w284:errorcluster)  [unwired: 8 in, 1 out]
        n206 = call "Corr Panel.vi"("error in"=w284, "adc session"=w274, "transducers in"=w276) -> ("error out"=w282:errorcluster, "adc session out"=w273:T14, "transducers out"=w275:T110)  [unwired: 6 in]
        n207 = Bundle By Name(cluster=w287, "corrections"=w275, "adc"=w273) -> (w286:T13)
        n208 = call "SGUI Set Control Enabled State By Groups.vi"("error in"=w282, "group name to enable (none)"="ready") -> ("error out"=w277:errorcluster)  [unwired: 8 in, 1 out]
        n209 = local write "session"(w286) -> ()
        n210 = call "GUI Set Error and Display Error Status.vi"("error in"=w277) -> ()  [unwired: 4 in]
      }
      event "qwtb maxarr", "qwtb res sel", "qwtb ref chn", "qwtb alg sel", "qwtb qu list", "qwtb save comment": Value Change {
        # "Result Viewer Update"
        n211 = event-data() -> ()  [unwired: 1 in, 6 out]
        n212 = call "Meas Proc QWTB Notify Result Queue.vi"("update comment (False)"="qwtb save comment") -> ("error out"=w289:errorcluster)  [unwired: 9 in, 1 out]
        n213 = call <vilib>:"Clear Errors.vi"("error in (no error)"=w289) -> ()  [unwired: 5 in, 2 out]
      }
      event "qwtb meas sel": Mouse Down {
        # "QWTB result viewer - changed measurement session"
        n214 = event-data() -> ()  [unwired: 1 in, 8 out]
        n215 = call "Meas Proc QWTB Notify Result Queue.vi"("new session? (False)"=TRUE) -> ("error out"=w291:errorcluster)  [unwired: 9 in, 1 out]
        n216 = call <vilib>:"Clear Errors.vi"("error in (no error)"=w291) -> ()  [unwired: 5 in, 2 out]
      }
      event "qwtb results table": Mouse Up {
        # "Update QWTB result selection"
        n217 = event-data() -> ("Mods"=w299:cluster{"Double Click":bool, "Menu Key":bool})  [unwired: 1 in, 7 out]
        n218 = control-ref of="qwtb results table"() -> (w292:refnum<vi>)
        n219 = local read "qwtb view"() -> (w294:T3)
        n220 = Unbundle By Name(w299) -> ("Double Click"=w298:bool)
        n221 = call "Meas Proc QWTB Fix Result Table Selection.vi"("param table ref"=w292) -> ("error out"=w293:errorcluster)  [unwired: 10 in]
        n222 = call "Meas Proc QWTB Set Result Table Sizes.vi"("param table ref"=w292, "error in"=w293) -> ("error out"=w296:errorcluster)  [unwired: 9 in]
        n223 = call "Meas Proc QWTB Update Result Table Variable Info.vi"("error in"=w296, "QWTB result session in"=w294) -> ("error out"=w295:errorcluster)  [unwired: 9 in]
        n224 = call <vilib>:"Clear Errors.vi"("error in (no error)"=w295) -> ("error out"=w297:errorcluster)  [unwired: 5 in, 1 out]
        n225 = case shown="True" w298 {
          selector: w298 -> [_ w304]
          tunnel: w297 -> [_ w301]
          frame False {
          }
          frame True {
            # "show graph"
            n226 = call "Meas Proc QWTB Result Plot Panel.vi"("error in"=w301) -> ("error out"=w303:errorcluster, "ok?"=w300:bool, "plot config"=w302:T119)  [unwired: 8 in]
            n227 = case shown="True" w300 {
              tunnel: [w306 w310] -> w305
              tunnel: w304 -> [_ w309]
              tunnel: w303 -> [w306 w308]
              tunnel: w302 -> [_ w307]
              frame False {
              }
              frame True {
                n228 = call "Meas Proc QWTB Notify Result Queue.vi"("plot setup"=w307, "error in"=w308, "show graph (False)"=w309) -> ("error out"=w310:errorcluster)  [unwired: 7 in, 1 out]
              }
            }
            n229 = call <vilib>:"Clear Errors.vi"("error in (no error)"=w305) -> ()  [unwired: 5 in, 2 out]
          }
        }
      }
      event "qwtb results table": Shortcut Menu Selection (User) {
        # "EXPORT QWTB RESULTS TABLE"
        n230 = event-data() -> ("ItemTag"=w311:string)  [unwired: 1 in, 7 out]
        n231 = case shown="\"raw session\"" w311 {
          selector: w311 -> [_ _ _ w340 _]
          frame Default {
          }
          frame "QWTB_TAB_SHOW_GRAPH" {
            # "SHOW GRAPH"
            n232 = local read "qwtb view"() -> (w317:T3)
            n233 = call "Meas Proc QWTB Update Result Table Variable Info.vi"("QWTB result session in"=w317) -> ("error out"=w318:errorcluster)  [unwired: 10 in]
            n234 = call <vilib>:"Clear Errors.vi"("error in (no error)"=w318) -> ("error out"=w316:errorcluster)  [unwired: 5 in, 1 out]
            n235 = call "Meas Proc QWTB Result Plot Panel.vi"("error in"=w316) -> ("error out"=w314:errorcluster, "ok?"=w312:bool, "plot config"=w313:T119)  [unwired: 8 in]
            n236 = case shown="True" w312 {
              tunnel: [w319 w323] -> w315
              tunnel: w314 -> [w319 w322]
              tunnel: w313 -> [_ w321]
              frame False {
              }
              frame True {
                n237 = call "Meas Proc QWTB Notify Result Queue.vi"("plot setup"=w321, "error in"=w322, "show graph (False)"=TRUE) -> ("error out"=w323:errorcluster)  [unwired: 7 in, 1 out]
              }
            }
            n238 = call <vilib>:"Clear Errors.vi"("error in (no error)"=w315) -> ()  [unwired: 5 in, 2 out]
          }
          frame "QWTB_TAB_CLOSE_GRAPHS" {
            # "Close all graphs"
            n239 = control-ref of="golpi"() -> (w326:refnum<vi>)
            n240 = call "golpi_mpc_get_access.vi"("golpi session ref"=w326) -> ("error out"=w331:errorcluster, "GOLPI ref out"=w329:T10, "golpi session ref out (copy)"=w327:T99)  [unwired: 5 in, 3 out]
            n241 = call "golpi_mpc_command.vi"("error in"=w331, "command"="close all;", "GOLPI ref in"=w329) -> ("error out"=w330:errorcluster, "GOLPI ref. out"=w328:T10)  [unwired: 6 in, 1 out]
            n242 = call "golpi_mpc_release.vi"("error in"=w330, "golpi ref or golpi session in"=w328, "golpi session ref"=w327) -> ("error out"=w324:errorcluster)  [unwired: 7 in, 1 out]
            n243 = call <vilib>:"Clear Errors.vi"("error in (no error)"=w324) -> ()  [unwired: 5 in, 2 out]
          }
          frame "QWTB_TAB_EXPORT_CLIP", "QWTB_TAB_EXPORT_XLS", "QWTB_TAB_EXPORT_XLS_ROW" {
            w352 = T122 {"Row"=0, "Column"=0} ("Selection Start")
            # "EXPORT TO EXCEL"
            n244 = property on="qwtb results table" class="Tbl (strict)"() -> (error out=w366:errorcluster, "Value"=w345:string[][], "Row Headers[]"=w361:string[], "Column Headers[]"=w360:string[])  [unwired: 2 in, 1 out]
            n245 = Equal?(x="QWTB_TAB_EXPORT_XLS_ROW", y=w340) -> (x = y?=w349:bool)
            n246 = local read "qwtb view"() -> (w344:T3)
            n247 = Transpose 2D Array(2D array=w345) -> (transposed array=w359:string[][])
            n248 = Build Array (concatenate)("", w360) -> (w357:string[])
            n249 = Build Array (concatenate)(w361, w359) -> (w367:string[][])
            n250 = Unbundle By Name(w344) -> ("matrix"=w343:dbl[][])
            n251 = Transpose 2D Array(2D array=w367) -> (transposed array=w358:string[][])
            n252 = Build Array (concatenate)(w357, w358) -> (w356:string[][])
            n253 = for {
              tunnel: [w384] -> w339 mode=indexing
              tunnel: w356 -> [w385] mode=indexing
              tunnel: w343 -> [w383] mode=indexing
              n254 = for {
                tunnel: [w390] -> w384 mode=indexing
                tunnel: w385 -> [w388] mode=indexing
                tunnel: w383 -> [w386] mode=indexing
                # "auto decimal sep."
                n255 = Not A Number/Path/Refnum?(number/path/refnum=w386) -> (NaN/Path/Refnum?=w389:bool)
                n256 = Format Into String(format string="%;%_9g", w386) -> (resulting string=w387:string)  [unwired: 2 in, 1 out]
                n257 = Select(t=w388, s=w389, f=w387) -> (s? t:f=w390:string)
              }
            }
            n258 = property on="qwtb results table" class="Tbl (strict)"() -> ("Selection Start"=w351:T122, "Selection Size"=w341:T122)  [unwired: 2 in, 2 out]
            n259 = Unbundle By Name(w351) -> ("Row"=w350:i32, "Column"=w342:i32)
            n260 = Unbundle By Name(w341) -> ("Row"=w333:i32, "Column"=w332:i32)
            n261 = Increment(x=w350) -> (x+1=w335:i32)
            n262 = Increment(x=w342) -> (x+1=w334:i32)
            n263 = Equal To 0?(x=w332) -> (x = 0?=w338:bool)
            n264 = Equal To 0?(x=w333) -> (x = 0?=w337:bool)
            n265 = Compound Arithmetic op=AND(w338, w337) -> (w336:bool)
            n266 = property on="exp tab" class="Tbl (strict)"(error in=w366, "Value"=w339) -> (error out=w365:errorcluster)  [unwired: 1 in, 1 out]
            n267 = Array Size(array=w339) -> (size(s)=w364:i32[])
            n268 = Bundle By Name(cluster=w352, "Row"=w335, "Column"=w334) -> (w353:T122)
            n269 = Array To Cluster(array=w364) -> (cluster=w346:cluster{"[0]":i32, "[1]":i32})
            n270 = Bundle By Name(cluster=w346, "[0]"=w333, "[1]"=w332) -> (w347:cluster{"[0]":i32, "[1]":i32})
            n271 = Select(t=w353, s=w349, f=w352) -> (s? t:f=w354:T122)
            n272 = Select(t=w347, s=w349, f=w346) -> (s? t:f=w348:cluster{"[0]":i32, "[1]":i32})
            n273 = property on="exp tab" class="Tbl (strict)"(error in=w365, "Selection Start"=w354, "Selection Size"=w348) -> (error out=w363:errorcluster)  [unwired: 1 in, 1 out]
            n274 = case shown="Default" w340 {
              tunnel: w363 -> [w378 w382]
              tunnel: w339 -> [w374 w379]
              tunnel: w336 -> [w375 _]
              tunnel: w335 -> [w371 _]
              tunnel: w334 -> [w370 _]
              tunnel: w333 -> [w369 _]
              tunnel: w332 -> [w368 _]
              frame "QWTB_TAB_EXPORT_CLIP" {
                n275 = Array Subset(array=w374, index (row)=w371, length (row)=w369, index (col)=w370, length (col)=w368) -> (w372:string[][])
                n276 = Select(t=w374, s=w375, f=w372) -> (s? t:f=w373:string[][])
                n277 = Array To Spreadsheet String(array=w373, 3:"%s" ("format string")) -> (spreadsheet string=w376:string)  [unwired: 1 in]
                n278 = invoke class="App" method="Clipboard.Write"(error in=w378, "Param 0"=w376) -> ()  [unwired: 2 in, 4 out]
              }
              frame Default {
                n279 = local read "qwtb view"() -> (w380:T3)
                n280 = call "Meas Proc QWTB Export Result.vi"("error in"=w382, "export data"=w379, "qwtb view"=w380) -> ("error out"=w381:errorcluster)  [unwired: 8 in]
                n281 = call "GUI Set Error and Display Error Status.vi"("error in"=w381) -> ()  [unwired: 4 in]
              }
            }
          }
          frame "raw session" {
            # "execute VI"
            # "open VI ref"
            # "VI to exec. prototype"
            # "get path of VI to execute"
            # "is reentrant?"
            # "call and forget mode"
            # "Show raw session INFO file"
            n282 = vi-ref "Text Viewer.vi"() -> (w394:refnum<vi>)
            n283 = local read "qwtb view"() -> (w408:T3)
            n284 = property class="VI"(reference=w394) -> (error out=w405:errorcluster, "Path"=w404:path, "Exec.IsReentrant"=w400:bool)  [unwired: 1 in, 1 out]
            n285 = Unbundle By Name(w408) -> ("last session"=w407:path)
            n286 = Select(t=64 ("options"), s=w400, f=0 ("options")) -> (s? t:f=w399:i32)
            n287 = Add(x=w399, y=128 ("options")) -> (x+y=w395:i32)
            n288 = Build Path(base path=w407, name or relative path="session.info") -> (appended path=w392:path)
            n289 = Open VI Reference(type specifier VI Refnum (for type only)=refnum<vi> refnum, vi path=w404, options=w395, error in (no error)=w405) -> (vi reference=w401:refnum<vi>, error out=w402:errorcluster)  [unwired: 2 in]
            n290 = call-by-ref "Start Asynchronous Call"(reference=w401, error in=w402, "Path"=w392) -> (error out=w393:errorcluster)  [unwired: 9 in, 3 out]
            n291 = call <vilib>:"Clear Errors.vi"("error in (no error)"=w393) -> ()  [unwired: 5 in, 2 out]
          }
        }
      }
      event "btn qwtb calc": Value Change {
        # "controls to ready state"
        # "clead error"
        # "write status info"
        # "set controls to busy state"
        # "invoke ADC configuration panel"
        # "Run QWTB batch processing panel"
        n292 = event-data() -> ()  [unwired: 1 in, 6 out]
        n293 = invoke on="error" class="Clust (strict)" method="Reinit To Default"() -> (error out=w417:errorcluster)  [unwired: 3 in, 2 out]
        n294 = call-poly "SGUI Assign String With Tags.vi"("error in"=w417, "label(s) (empty)"="stat1" ("control label (none)"), "string (empty)"="<tc=gold><b>QWTB batch processing...") -> ("error out"=w416:errorcluster)  [unwired: 7 in, 1 out]
        n295 = call "SGUI Set Control Enabled State By Groups.vi"("error in"=w416, "group name to enable (none)"="busy") -> ("error out"=w412:errorcluster)  [unwired: 8 in, 1 out]
        n296 = local read "session"() -> (w410:T13)
        n297 = call "Meas Batch Proc QWTB Panel.vi"("error in"=w412, "session in"=w410) -> ("error out"=w411:errorcluster, "session out"=w409:T13)  [unwired: 8 in]
        n298 = local write "session"(w409) -> ()
        n299 = call "SGUI Set Control Enabled State By Groups.vi"("error in"=w411, "group name to enable (none)"="ready") -> ("error out"=w413:errorcluster)  [unwired: 8 in, 1 out]
        n300 = call "GUI Set Error and Display Error Status.vi"("error in"=w413) -> ()  [unwired: 4 in]
      }
      event "btn srv": Value Change {
        # "Start TWM server"
        n301 = event-data() -> ()  [unwired: 1 in, 6 out]
        n302 = invoke on="error" class="Clust (strict)" method="Reinit To Default"() -> (error out=w422:errorcluster)  [unwired: 3 in, 2 out]
        n303 = control-ref of="server"() -> (w421:refnum<vi>)
        n304 = vi-ref "Server Panel.vi"() -> (w424:refnum<vi>)
        n305 = To Variant(anything=w421) -> (Variant=w425:variant)
        n306 = call "Meas Asynchronous Start.vi"("error in"=w422, "parameter in"=w425, "Static VI reference in (empty)"=w424) -> ("error out"=w420:errorcluster, "async VI reference out"=w423:refnum<vi>)  [unwired: 7 in]
        n307 = local write "server vi ref"(w423) -> ()
        n308 = call "GUI Set Error and Display Error Status.vi"("error in"=w420) -> ()  [unwired: 4 in]
        n309 = case shown="No Error" w420 {
          frame No Error {
            n310 = call "SGUI Set Control Enabled State By Label.vi"("labels (empty)"="btn srv", "Enabled? (False)"=FALSE) -> ()  [unwired: 8 in, 2 out]
          }
          frame Error {
          }
        }
      }
      event User Event {
        # "SERVER COMMANDS EVENT HANDLER"
        n311 = event-data() -> ("client request"=w430:T117, "command"=w431:T115)  [unwired: 1 in, 4 out]
        n312 = property on="btn stop" class="Bool (strict)"() -> (error out=w429:errorcluster, "DisabledEnum"=w428:T118)  [unwired: 2 in, 1 out]
        n313 = case shown="\"Get status\"" w431 {
          tunnel: w430 -> [_ w434 _ _ _ _ w551 w580 w597 w612 w631 w650 _]
          tunnel: w429 -> [_ w433 w454 w512 w533 w539 w549 w578 w595 w614 w633 w652 w670]
          tunnel: w428 -> [_ w432 w455 w511 w534 w540 w550 w579 w596 w613 w632 w651 w669]
          frame Default {
          }
          frame "Set measurement" {
            n314 = case shown="\"Disabled and Grayed Out\"" w432 {
              tunnel: w434 -> [_ w443]
              tunnel: w433 -> [_ w436]
              frame Default {
              }
              frame "Disabled and Grayed Out" {
                # "send ACK"
                # "no GUI"
                # "parse and set\nsampling and\nprocessing parameters"
                # "controls ready"
                # "invoke config panel or config\nvalidity check\n\nnote: here in server mode\nit will just regenerate sequence\nand check destination path"
                # "update status"
                # "controls busy"
                n315 = invoke on="error" class="Clust (strict)" method="Reinit To Default"(error in=w436) -> (error out=w449:errorcluster)  [unwired: 2 in, 2 out]
                n316 = call-poly "SGUI Assign String With Tags.vi"("error in"=w449, "label(s) (empty)"="stat1\nstat2\nstat3", "string (empty)"="<tc=gold><b>TWM server - Setting new measurement...\n\n") -> ("error out"=w448:errorcluster)  [unwired: 7 in, 1 out]
                n317 = call "SGUI Set Control Enabled State By Groups.vi"("error in"=w448, "group name to enable (none)"="busy") -> ("error out"=w446:errorcluster)  [unwired: 8 in, 1 out]
                n318 = local read "session"() -> (w445:T13)
                n319 = call "Server Cmd Parser - Set Measurement.vi"("error in"=w446, "client request"=w443, "session in"=w445) -> ("error out"=w444:errorcluster, "session out"=w438:T13)  [unwired: 7 in]
                n320 = call "Meas Config Panel.vi"("error in"=w444, "force no GUI (False)"=TRUE, "session in"=w438) -> ("error out"=w435:errorcluster, "session out"=w437:T13)  [unwired: 6 in, 1 out]
                n321 = local write "session"(w437) -> ()
                n322 = control-ref of="server"() -> (w440:refnum<vi>)
                n323 = call "Server Generate ACK Event.vi"("error data to send (in error case)"=w435, "error in"=w435, "header"="Set measurement" ("event data"), "server event ref"=w440) -> ("error out"=w441:errorcluster)  [unwired: 7 in]
                n324 = call "SGUI Set Control Enabled State By Groups.vi"("error in"=w441, "group name to enable (none)"="ready") -> ("error out"=w451:errorcluster)  [unwired: 8 in, 1 out]
                n325 = call "GUI Set Error and Display Error Status.vi"("error in"=w451) -> ()  [unwired: 4 in]
              }
            }
          }
          frame "Start" {
            n326 = case shown="\"Disabled and Grayed Out\"" w455 {
              tunnel: w454 -> [_ w457]
              frame Default {
              }
              frame "Disabled and Grayed Out" {
                # "server command?"
                # "invoke config\npanel or config\nvalidity check"
                # "start measurement"
                # "update status"
                # "controls busy"
                n327 = local read "start btns"() -> (w466:T2)
                n328 = Unbundle By Name(w466) -> ("start"=w465:bool, "setup"=w464:bool, "setup&start"=w463:bool)
                n329 = invoke on="error" class="Clust (strict)" method="Reinit To Default"(error in=w457) -> (error out=w478:errorcluster)  [unwired: 2 in, 2 out]
                n330 = Compound Arithmetic op=OR(w463, w464, w465) -> (invert w460:bool)
                n331 = flat-sequence {
                  tunnel: w460 -> [_]
                  frame #0 {
                    n332 = local write "start btns"(T2 {"start"=FALSE, "setup"=FALSE, "setup&start"=FALSE} ("start btns")) -> ()
                  }
                }
                n333 = call-poly "SGUI Assign String With Tags.vi"("error in"=w478, "label(s) (empty)"="stat1\nstat2\nstat3", "string (empty)"="<tc=gold><b>Starting measurement...\n\n") -> ("error out"=w477:errorcluster)  [unwired: 7 in, 1 out]
                n334 = call "SGUI Set Control Enabled State By Groups.vi"("error in"=w477, "group name to enable (none)"="busy") -> ("error out"=w474:errorcluster)  [unwired: 8 in, 1 out]
                n335 = local read "session"() -> (w459:T13)
                n336 = Compound Arithmetic op=OR(w464, w463) -> (w468:bool)
                n337 = call "Meas Config Panel.vi"("error in"=w474, "force no GUI (False)"=w460, "always show setup (False)"=w468, "session in"=w459) -> ("error out"=w473:errorcluster, "canceled?"=w470:bool, "session out"=w458:T13)  [unwired: 5 in]
                n338 = Compound Arithmetic op=OR(w460, w465, w463) -> (w467:bool)
                n339 = Compound Arithmetic op=AND(w467, invert w470) -> (invert w469:bool)
                n340 = case shown="False" w469 {
                  tunnel: [w501 _] -> w475
                  tunnel: w473 -> [w498 w504]
                  tunnel: w458 -> [w493 w503]
                  tunnel: [w500 w504] -> w471
                  tunnel: [w494 w503] -> w456
                  frame False {
                    # "digitizer busy"
                    n341 = Unbundle By Name(w493) -> ("adc"=w499:T14)
                    n342 = Unbundle By Name(w493) -> ("sequence"=w492:T93[])
                    n343 = call "ADC Reset Idle Timer.vi"("error in"=w498, "set busy (False)"=TRUE, "adc session in"=w499) -> ("error out"=w496:errorcluster, "adc session out"=w497:T14)  [unwired: 7 in]
                    n344 = Index Array(array=w492) -> (element=w491:T93)  [unwired: 1 in]
                    n345 = Bundle By Name(cluster=w493, "adc"=w497) -> (w494:T13)
                    n346 = local read "qwtb view"() -> (w490:T3)
                    n347 = Unbundle By Name(w491) -> ("meas root path"=w488:path)
                    n348 = Bundle By Name(cluster=w490, "last session"=w488) -> (w489:T3)
                    n349 = local write "qwtb view"(w489) -> ()
                    n350 = vi-ref "Meas Main.vi"() -> (w502:refnum<vi>)
                    n351 = call "Meas Asynchronous Start.vi"("error in"=w496, "parameter in"=w494, "Static VI reference in (empty)"=w502) -> ("error out"=w500:errorcluster, "async VI reference out"=w501:refnum<vi>)  [unwired: 7 in]
                  }
                  frame True {
                  }
                }
                n352 = local write "session"(w456) -> ()
                n353 = Compound Arithmetic op=OR(w471, w469) -> (w472:bool)
                n354 = case shown="True" w472 {
                  tunnel: [w506 w509] -> w462
                  tunnel: [TRUE _] -> w480
                  tunnel: w475 -> [w507 _]
                  tunnel: w471 -> [w506 w508]
                  frame False {
                    # "success, remember\nsession VI reference"
                    n355 = local write "session VI ref"(w507) -> ()
                  }
                  frame True {
                    # "controls ready"
                    # "async start failed\nrestore controls"
                    n356 = call "SGUI Set Control Enabled State By Groups.vi"("error in"=w508, "group name to enable (none)"="ready") -> ("error out"=w509:errorcluster)  [unwired: 8 in, 1 out]
                  }
                }
                n357 = case shown="True" w460 {
                  tunnel: w462 -> [w483 w484]
                  tunnel: [w483 w486] -> w461
                  frame False {
                  }
                  frame True {
                    # "Server ACK"
                    n358 = control-ref of="server"() -> (w487:refnum<vi>)
                    n359 = call "Server Generate ACK Event.vi"("error data to send (in error case)"=w484, "error in"=w484, "header"="Start", "server event ref"=w487) -> ("error out"=w486:errorcluster)  [unwired: 7 in]
                  }
                }
                n360 = call "GUI Set Error and Display Error Status.vi"("error in"=w461, "Write status only if error occures? (False)"=w480) -> ()  [unwired: 3 in]
              }
            }
          }
          frame "Identify" {
            n361 = case shown="\"Disabled and Grayed Out\"" w511 {
              tunnel: w512 -> [_ w513]
              frame Default {
              }
              frame "Disabled and Grayed Out" {
                # "identify instruments"
                # "controls ready"
                # "update status"
                # "controls busy"
                n362 = invoke on="error" class="Clust (strict)" method="Reinit To Default"(error in=w513) -> (error out=w526:errorcluster)  [unwired: 2 in, 2 out]
                n363 = call-poly "SGUI Assign String With Tags.vi"("error in"=w526, "label(s) (empty)"="stat1\nstat2\nstat3", "string (empty)"="<tc=gold><b>TWM server - Identification of instruments...\n\n") -> ("error out"=w525:errorcluster)  [unwired: 7 in, 1 out]
                n364 = call "SGUI Set Control Enabled State By Groups.vi"("error in"=w525, "group name to enable (none)"="busy") -> ("error out"=w523:errorcluster)  [unwired: 8 in, 1 out]
                n365 = local read "session"() -> (w521:T13)
                n366 = Unbundle By Name(w521) -> ("adc"=w522:T14)
                n367 = call "ADC Get Capabilities.vi"("Initialize HW? (False)"=TRUE, "error in"=w523, "adc session in"=w522) -> ("error out"=w518:errorcluster, "adc session out"=w516:T14)  [unwired: 6 in, 1 out]
                n368 = Bundle By Name(cluster=w521, "adc"=w516) -> (w520:T13)
                n369 = local write "session"(w520) -> ()
                n370 = control-ref of="server"() -> (w517:refnum<vi>)
                n371 = call "Server Cmd Answer - Identify.vi"("server event ref"=w517, "error in"=w518, "command header (none)"="Identify", "adc session"=w516) -> ("error out"=w519:errorcluster)  [unwired: 6 in, 1 out]
                n372 = call "SGUI Set Control Enabled State By Groups.vi"("error in"=w519, "group name to enable (none)"="ready") -> ("error out"=w528:errorcluster)  [unwired: 8 in, 1 out]
                n373 = call "GUI Set Error and Display Error Status.vi"("error in"=w528) -> ()  [unwired: 4 in]
              }
            }
          }
          frame "Get status" {
            # "last error (hopefully upadated at this point)"
            # "is ready?"
            n374 = Equal?(x=w534, y=T118."Disabled and Grayed Out") -> (x = y?=w535:bool)
            n375 = local read "error"() -> (w532:errorcluster)
            n376 = control-ref of="server"() -> (w536:refnum<vi>)
            n377 = call "Server Cmd Answer - Get Status.vi"("error message in"=w532, "server event ref"=w536, "error in"=w533, "Status ready? (False)"=w535) -> ("error out"=w537:errorcluster, "error message out"=w531:errorcluster)  [unwired: 5 in, 1 out]
            n378 = local write "error"(w531) -> ()
            n379 = call <vilib>:"Clear Errors.vi"("error in (no error)"=w537) -> ()  [unwired: 5 in, 2 out]
          }
          frame "Stop" {
            # "send ACK"
            # "Set STOP state if running"
            n380 = case shown="\"Enabled\"" w540 {
              tunnel: w539 -> [w545 w547]
              tunnel: [w545 w546] -> w544
              frame Default {
              }
              frame "Enabled" {
                n381 = property on="btn stop" class="Bool (strict)"(error in=w547, "Val(Sgnl)"=TRUE ("Value (Signaling)")) -> (error out=w546:errorcluster)  [unwired: 1 in, 1 out]
              }
            }
            n382 = control-ref of="server"() -> (w543:refnum<vi>)
            n383 = call "Server Generate ACK Event.vi"("error in"=w544, "header"="Stop", "server event ref"=w543) -> ("error out"=w541:errorcluster)  [unwired: 8 in]
            n384 = call <vilib>:"Clear Errors.vi"("error in (no error)"=w541) -> ()  [unwired: 5 in, 2 out]
          }
          frame "Set corrections" {
            n385 = case shown="\"Disabled and Grayed Out\"" w550 {
              tunnel: w551 -> [_ w576]
              tunnel: w549 -> [_ w556]
              frame Default {
              }
              frame "Disabled and Grayed Out" {
                w571 = "" ("status name label")
                # "send ACK"
                # "update status"
                # "controls busy"
                n386 = invoke on="error" class="Clust (strict)" method="Reinit To Default"(error in=w556) -> (error out=w562:errorcluster)  [unwired: 2 in, 2 out]
                n387 = call-poly "SGUI Assign String With Tags.vi"("error in"=w562, "label(s) (empty)"="stat1\nstat2\nstat3", "string (empty)"="<tc=gold><b>TWM server - Setting corrections...\n\n") -> ("error out"=w561:errorcluster)  [unwired: 7 in, 1 out]
                n388 = call "SGUI Set Control Enabled State By Groups.vi"("error in"=w561, "group name to enable (none)"="busy") -> ("error out"=w559:errorcluster)  [unwired: 8 in, 1 out]
                n389 = local read "session"() -> (w577:T13)
                n390 = call "Server Cmd Parser - Set Corrections.vi"("error in"=w559, "client request"=w576, "session in"=w577) -> ("error out"=w572:errorcluster, "session out"=w568:T13)  [unwired: 7 in]
                n391 = Unbundle By Name(w568) -> ("corrections.transducers"=w575:T123, "corrections.digitizer"=w574:T112, "adc"=w573:T14)
                n392 = call "Corr Transducers Reload All.vi"("error in"=w572, "transducers in"=w575) -> ("error out"=w570:errorcluster, "transducers out"=w567:T123)  [unwired: 5 in, 3 out]
                n393 = call "Corr Digitizer Check.vi"("correction path label"=w571, "status name label"=w571, "correction name label"=w571, "error in"=w572, "adc session"=w573, "digitizer corrections in"=w574) -> ("error out"=w569:errorcluster, "digitizer corrections out"=w566:T112)  [unwired: 2 in, 2 out]
                n394 = Bundle By Name(cluster=w568, "corrections.transducers"=w567, "corrections.digitizer"=w566) -> (w565:T13)
                n395 = Merge Errors(w570, w569) -> (w552:errorcluster)
                n396 = local write "session"(w565) -> ()
                n397 = control-ref of="server"() -> (w555:refnum<vi>)
                n398 = call "Server Generate ACK Event.vi"("error data to send (in error case)"=w552, "error in"=w552, "header"="Set corrections" ("event data"), "server event ref"=w555) -> ("error out"=w553:errorcluster)  [unwired: 7 in]
                n399 = call "SGUI Set Control Enabled State By Groups.vi"("error in"=w553, "group name to enable (none)"="ready") -> ("error out"=w557:errorcluster)  [unwired: 8 in, 1 out]
                n400 = call "GUI Set Error and Display Error Status.vi"("error in"=w557) -> ()  [unwired: 4 in]
              }
            }
          }
          frame "Get result" {
            n401 = case shown="\"Disabled and Grayed Out\"" w579 {
              tunnel: w580 -> [_ w584]
              tunnel: w578 -> [_ w581]
              frame Default {
              }
              frame "Disabled and Grayed Out" {
                n402 = invoke on="error" class="Clust (strict)" method="Reinit To Default"(error in=w581) -> (error out=w592:errorcluster)  [unwired: 2 in, 2 out]
                n403 = call-poly "SGUI Assign String With Tags.vi"("error in"=w592, "label(s) (empty)"="stat1\nstat2\nstat3", "string (empty)"="<tc=gold><b>TWM server - Reading results...\n\n") -> ("error out"=w591:errorcluster)  [unwired: 7 in, 1 out]
                n404 = call "SGUI Set Control Enabled State By Groups.vi"("error in"=w591, "group name to enable (none)"="busy") -> ("error out"=w587:errorcluster)  [unwired: 8 in, 1 out]
                n405 = local read "session"() -> (w586:T13)
                n406 = control-ref of="server"() -> (w582:refnum<vi>)
                n407 = call "Server Cmd Answer - Get Result.vi"("server event ref"=w582, "error in"=w587, "client request"=w584, "session in"=w586) -> ("error out"=w583:errorcluster, "session out"=w585:T13)  [unwired: 6 in]
                n408 = local write "session"(w585) -> ()
                n409 = call "SGUI Set Control Enabled State By Groups.vi"("error in"=w583, "group name to enable (none)"="ready") -> ("error out"=w588:errorcluster)  [unwired: 8 in, 1 out]
                n410 = call "GUI Set Error and Display Error Status.vi"("error in"=w588) -> ()  [unwired: 4 in]
              }
            }
          }
          frame "Get algorithm info" {
            n411 = case shown="\"Disabled and Grayed Out\"" w596 {
              tunnel: w597 -> [_ w601]
              tunnel: w595 -> [_ w598]
              frame Default {
              }
              frame "Disabled and Grayed Out" {
                n412 = invoke on="error" class="Clust (strict)" method="Reinit To Default"(error in=w598) -> (error out=w609:errorcluster)  [unwired: 2 in, 2 out]
                n413 = call-poly "SGUI Assign String With Tags.vi"("error in"=w609, "label(s) (empty)"="stat1\nstat2\nstat3", "string (empty)"="<tc=gold><b>TWM server - Get algorithm info...\n\n") -> ("error out"=w608:errorcluster)  [unwired: 7 in, 1 out]
                n414 = call "SGUI Set Control Enabled State By Groups.vi"("error in"=w608, "group name to enable (none)"="busy") -> ("error out"=w604:errorcluster)  [unwired: 8 in, 1 out]
                n415 = local read "session"() -> (w603:T13)
                n416 = control-ref of="server"() -> (w599:refnum<vi>)
                n417 = call "Server Cmd Answer - Get Algorithm Info.vi"("server event ref"=w599, "error in"=w604, "client request"=w601, "session in"=w603) -> ("error out"=w600:errorcluster, "session out"=w602:T13)  [unwired: 6 in]
                n418 = local write "session"(w602) -> ()
                n419 = call "SGUI Set Control Enabled State By Groups.vi"("error in"=w600, "group name to enable (none)"="ready") -> ("error out"=w605:errorcluster)  [unwired: 8 in, 1 out]
                n420 = call "GUI Set Error and Display Error Status.vi"("error in"=w605) -> ()  [unwired: 4 in]
              }
            }
          }
          frame "Define Multiplexer Paths" {
            n421 = case shown="\"Disabled and Grayed Out\"" w613 {
              tunnel: w614 -> [_ w623]
              tunnel: w612 -> [_ w615]
              frame Default {
              }
              frame "Disabled and Grayed Out" {
                # "ACK"
                # "controls ready"
                # "update status"
                # "controls busy"
                n422 = invoke on="error" class="Clust (strict)" method="Reinit To Default"(error in=w623) -> (error out=w626:errorcluster)  [unwired: 2 in, 2 out]
                n423 = call-poly "SGUI Assign String With Tags.vi"("error in"=w626, "label(s) (empty)"="stat1\nstat2\nstat3", "string (empty)"="<tc=gold><b>Defining multiplexer paths ...\n\n") -> ("error out"=w625:errorcluster)  [unwired: 7 in, 1 out]
                n424 = call "SGUI Set Control Enabled State By Groups.vi"("error in"=w625, "group name to enable (none)"="busy") -> ("error out"=w620:errorcluster)  [unwired: 8 in, 1 out]
                n425 = local read "session"() -> (w618:T13)
                n426 = call "Server Cmd Parser - Define Multiplex Paths.vi"("error in"=w620, "client request"=w615, "session in"=w618) -> ("error out"=w619:errorcluster, "session out"=w617:T13)  [unwired: 7 in]
                n427 = local write "session"(w617) -> ()
                n428 = control-ref of="server"() -> (w622:refnum<vi>)
                n429 = call "Server Generate ACK Event.vi"("error data to send (in error case)"=w619, "error in"=w619, "header"="Define Multiplexer Paths", "server event ref"=w622) -> ("error out"=w621:errorcluster)  [unwired: 7 in]
                n430 = call "SGUI Set Control Enabled State By Groups.vi"("error in"=w621, "group name to enable (none)"="ready") -> ("error out"=w628:errorcluster)  [unwired: 8 in, 1 out]
                n431 = call "GUI Set Error and Display Error Status.vi"("error in"=w628) -> ()  [unwired: 4 in]
              }
            }
          }
          frame "Define QPMX" {
            n432 = case shown="\"Disabled and Grayed Out\"" w632 {
              tunnel: w633 -> [_ w642]
              tunnel: w631 -> [_ w634]
              frame Default {
              }
              frame "Disabled and Grayed Out" {
                # "ACK"
                # "controls ready"
                # "update status"
                # "controls busy"
                n433 = invoke on="error" class="Clust (strict)" method="Reinit To Default"(error in=w642) -> (error out=w645:errorcluster)  [unwired: 2 in, 2 out]
                n434 = call-poly "SGUI Assign String With Tags.vi"("error in"=w645, "label(s) (empty)"="stat1\nstat2\nstat3", "string (empty)"="<tc=gold><b>Defining QPMX paths ...\n\n") -> ("error out"=w644:errorcluster)  [unwired: 7 in, 1 out]
                n435 = call "SGUI Set Control Enabled State By Groups.vi"("error in"=w644, "group name to enable (none)"="busy") -> ("error out"=w638:errorcluster)  [unwired: 8 in, 1 out]
                n436 = local read "session"() -> (w635:T13)
                n437 = call "Server Cmd Parser - Define QPMX.vi"("error in"=w638, "client request"=w634, "session in"=w635) -> ("error out"=w637:errorcluster, "session out"=w636:T13)  [unwired: 7 in]
                n438 = local write "session"(w636) -> ()
                n439 = control-ref of="server"() -> (w641:refnum<vi>)
                n440 = call "Server Generate ACK Event.vi"("error data to send (in error case)"=w637, "error in"=w637, "header"="Define QPMX", "server event ref"=w641) -> ("error out"=w640:errorcluster)  [unwired: 7 in]
                n441 = call "SGUI Set Control Enabled State By Groups.vi"("error in"=w640, "group name to enable (none)"="ready") -> ("error out"=w647:errorcluster)  [unwired: 8 in, 1 out]
                n442 = call "GUI Set Error and Display Error Status.vi"("error in"=w647) -> ()  [unwired: 4 in]
              }
            }
          }
          frame "Define Multiplexer Sequence" {
            n443 = case shown="\"Disabled and Grayed Out\"" w651 {
              tunnel: w652 -> [_ w661]
              tunnel: w650 -> [_ w653]
              frame Default {
              }
              frame "Disabled and Grayed Out" {
                # "ACK"
                # "controls ready"
                # "update status"
                # "controls busy"
                n444 = invoke on="error" class="Clust (strict)" method="Reinit To Default"(error in=w661) -> (error out=w664:errorcluster)  [unwired: 2 in, 2 out]
                n445 = call-poly "SGUI Assign String With Tags.vi"("error in"=w664, "label(s) (empty)"="stat1\nstat2\nstat3", "string (empty)"="<tc=gold><b>Defining multiplexer sequence ...\n\n") -> ("error out"=w663:errorcluster)  [unwired: 7 in, 1 out]
                n446 = call "SGUI Set Control Enabled State By Groups.vi"("error in"=w663, "group name to enable (none)"="busy") -> ("error out"=w658:errorcluster)  [unwired: 8 in, 1 out]
                n447 = local read "session"() -> (w656:T13)
                n448 = call "Server Cmd Parser - Define Multiplex Sequence.vi"("error in"=w658, "client request"=w653, "session in"=w656) -> ("error out"=w657:errorcluster, "session out"=w655:T13)  [unwired: 7 in]
                n449 = local write "session"(w655) -> ()
                n450 = control-ref of="server"() -> (w660:refnum<vi>)
                n451 = call "Server Generate ACK Event.vi"("error data to send (in error case)"=w657, "error in"=w657, "header"="Define Multiplexer Sequence", "server event ref"=w660) -> ("error out"=w659:errorcluster)  [unwired: 7 in]
                n452 = call "SGUI Set Control Enabled State By Groups.vi"("error in"=w659, "group name to enable (none)"="ready") -> ("error out"=w666:errorcluster)  [unwired: 8 in, 1 out]
                n453 = call "GUI Set Error and Display Error Status.vi"("error in"=w666) -> ()  [unwired: 4 in]
              }
            }
          }
          frame "ADC selfcal" {
            n454 = case shown="\"Disabled and Grayed Out\"" w669 {
              tunnel: w670 -> [_ w676]
              frame Default {
              }
              frame "Disabled and Grayed Out" {
                # "ACK"
                # "run selfcal without GUI"
                # "controls ready"
                # "update status"
                # "controls busy"
                n455 = invoke on="error" class="Clust (strict)" method="Reinit To Default"(error in=w676) -> (error out=w684:errorcluster)  [unwired: 2 in, 2 out]
                n456 = call-poly "SGUI Assign String With Tags.vi"("error in"=w684, "label(s) (empty)"="stat1\nstat2\nstat3", "string (empty)"="<tc=gold><b>TWM server - Self-calibration of digitizer(s)...\n\n") -> ("error out"=w683:errorcluster)  [unwired: 7 in, 1 out]
                n457 = call "SGUI Set Control Enabled State By Groups.vi"("error in"=w683, "group name to enable (none)"="busy") -> ("error out"=w681:errorcluster)  [unwired: 8 in, 1 out]
                n458 = local read "session"() -> (w679:T13)
                n459 = Unbundle By Name(w679) -> ("adc"=w680:T14)
                n460 = call "ADC Selfcal Virtual Channels.vi"("error in"=w681, "Ignore GUI, force selfcal (False)"=TRUE ("Initialize HW? (False)"), "adc session in"=w680) -> ("error out"=w673:errorcluster, "adc session out"=w677:T14)  [unwired: 7 in]
                n461 = Bundle By Name(cluster=w679, "adc"=w677) -> (w678:T13)
                n462 = local write "session"(w678) -> ()
                n463 = control-ref of="server"() -> (w674:refnum<vi>)
                n464 = call "Server Generate ACK Event.vi"("error data to send (in error case)"=w673, "error in"=w673, "header"="ADC selfcal" ("command header (none)"), "server event ref"=w674) -> ("error out"=w671:errorcluster)  [unwired: 7 in]
                n465 = call "SGUI Set Control Enabled State By Groups.vi"("error in"=w671, "group name to enable (none)"="ready") -> ("error out"=w686:errorcluster)  [unwired: 8 in, 1 out]
                n466 = call "GUI Set Error and Display Error Status.vi"("error in"=w686) -> ()  [unwired: 4 in]
              }
            }
          }
        }
      }
      event Pane Size {
        # "Panel scaling layout - manual, because LV native scaling with pane in pain..."
        n467 = event-data() -> ()  [unwired: 1 in, 6 out]
        n468 = vi-ref "main.vi"() -> (w691:refnum<vi>)
        n469 = call "Scale Controls Helper.vi"("Action (Initialize)"=enum16{"Initialize", "Resize", "Resize?"}."Resize", "vi reference"=w691) -> ("error out"=w690:errorcluster)  [unwired: 9 in]
        n470 = call <vilib>:"Clear Errors.vi"("error in (no error)"=w690) -> ()  [unwired: 5 in, 2 out]
      }
    }
  }
